vi "Example.vi"() -> ()   [LabVIEW 2016]
uses:
  Controls/Init_Parameters.ctl
  Controls/Error_Out.ctl
  Controls/ActorScalingDetailsLowT_Parameters.ctl
  Controls/ActorScalingDetailsRoomT_Parameters.ctl
  Controls/Frequency-Control_Parameters.ctl
  Controls/Actual-Value_Selection.ctl
  Controls/Invert-Polarity_Selection.ctl
  Controls/Amplitude-Control_Parameters.ctl
  Controls/Autoapproach_Parameters.ctl
  Controls/Stop-Condition-Autoapproach_Selection.ctl
  Controls/Autoapproach-Approach-Mode_Selection.ctl
  Controls/Autoapproach-Target-Mode_Selection.ctl
  Controls/Autoapproach-Details_Parameters.ctl
  Controls/Autoapproach-Axis_Selection.ctl
  Controls/Appraoch-Direction_Selection.ctl
  Controls/Autoapproach-Device_Selection.ctl
  Controls/Autoapproach-Trigger_Selection.ctl
  Controls/Ground-while-Appraoch_Selection.ctl
  Controls/DAC_Selection.ctl
  Controls/Generic-Feedback_Parameters.ctl
  Controls/Generic-Feedback-Number_Selection.ctl
  Controls/Generic-Feedback-Input-Channel_Selection.ctl
  Controls/Generic-Feedback-Output-Channel_Selection.ctl
  Controls/LF-Lockin_Parameters.ctl
  Controls/LF-Lockin-Output-Connector_Selection.ctl
  Controls/LF-Lockin-Input-Connector_Selection.ctl
  Controls/HF-Lockin_Parameters.ctl
  Controls/External-Transfer-Function_Parameters.ctl
  Controls/External-Transfer-Function_Selection.ctl
  Controls/External-Transfer-Function-Unit_Selection.ctl
  Controls/Dual-Pass_Parameters.ctl
  Controls/Dual-Pass-Alternative-Setpoint_Selection.ctl
  Controls/Dual-Pass-Alternative-DAC_Selection.ctl
  Controls/Dual-Pass-Alternative-Fexc_Selection.ctl
  Controls/Dual-Pass-Feedback-Mode_Selection.ctl
  Controls/Dual-Pass-State_Selection.ctl
  Controls/Scan_Parameters.ctl
  Controls/Spectroscopy_Parameters.ctl
  Controls/Spectroscopy-Mode_Selection.ctl
  Controls/Spec_DAC_Selection.ctl
  Controls/Channel_Parameters.ctl
  Controls/Channel_Selection.ctl
  Controls/Channel-Source_Selection.ctl
  Controls/Average_Selection.ctl
  Controls/Trigger_Selection.ctl
  Controls/Pathmode_Parameters.ctl
  Controls/Path-Mode-Edge_Selection.ctl
  Controls/Pathmode-Action_Selection.ctl
  Controls/Scanner_State_Machine.ctl
  Controls/DAC_Voltage.ctl
  Controls/DAC_Limits.ctl
  Controls/Z-Control_Parameters.ctl
  Controls/Coarse-Axis_Selection.ctl
  Controls/Grid_Parameters.ctl
  Controls/Output-Activation_Selection.ctl
panel:
  out "ScanUnits":string[](array[string])
  in  "Z Control Cluster":T1={"Input Signal"=0, "Min"=-inf, "Max"=-inf, "P"=-inf, "Setpoint a.u."=-inf, "Invert Polarity"=-2147483648, "I"=-inf} {"I" format="%#_g mHz"; "Invert Polarity" items=["[read only]"=-2147483648, "No"=0, "Yes"=1]; "Max" format="%#_g nm"; "Min" format="%#_g nm"; "Input Signal" items=["[read only]"=-2147483648, "ADC 1"=0, "ADC 2"=1, "ADC 3"=2, "ADC 4"=3, "ADC 5"=4, "ADC 6"=5, "HF 1 df"=8, "HF 1 Ampl"=13, "HF 1 Phase"=14, "LockIn Ampl"=16, "LockIn Phase"=17, "Counter"=23]}
  in  "Use sensor position":bool
  out "ErrCrt_Spec":bool
  out "ErrCrt_Line":bool
  out "storage paths":string[](array[string])
  in  "ScanStop":bool
  in  "Environment Temperature":sgl(slide)
  out "Enum":T4
  in  "Name of Profile":string="afm.ngp"
  in  "loop wait":u32=100 format="%.0f ms"
  out "unit_val 3":T5=-2147483648 items=["[read only]"=-2147483648, "Not Valid"=128, "m"=384, "mm"=383, "um"=382, "nm"=381, "pm"=380, "V"=640, "mV"=639, "uV"=638, "nV"=637, "MHz"=898, "kHz"=897, "Hz"=896, "mHz"=895, "Ks"=1153, "s"=1152, "ms"=1151, "us"=1150, "ns"=1149, "ps"=1148, "A"=1408, "mA"=1407, "uA"=1406, "nA"=1405, "W"=1664, "mW"=1663, "uW"=1662, "nW"=1661, "T"=1920, "mT"=1919, "uT"=1918, "nT"=1917, "K"=2176, "mK"=2175, "uK"=2174, "nK"=2173, "Deg"=2432, "mDeg"=2431, "uDeg"=2430, "nDeg"=2429, "[cos]"=2688, "[dB]"=2944, "LSB"=3200]
  out "unit_xy 3":T5=-2147483648 items=["[read only]"=-2147483648, "Not Valid"=128, "m"=384, "mm"=383, "um"=382, "nm"=381, "pm"=380, "V"=640, "mV"=639, "uV"=638, "nV"=637, "MHz"=898, "kHz"=897, "Hz"=896, "mHz"=895, "Ks"=1153, "s"=1152, "ms"=1151, "us"=1150, "ns"=1149, "ps"=1148, "A"=1408, "mA"=1407, "uA"=1406, "nA"=1405, "W"=1664, "mW"=1663, "uW"=1662, "nW"=1661, "T"=1920, "mT"=1919, "uT"=1918, "nT"=1917, "K"=2176, "mK"=2175, "uK"=2174, "nK"=2173, "Deg"=2432, "mDeg"=2431, "uDeg"=2430, "nDeg"=2429, "[cos]"=2688, "[dB]"=2944, "LSB"=3200]
  out "Intensity Graph":sgl[][](graph)
  out "ErrorStop":bool
  out "ErrCrt_Scan":bool
  out "unit_val":T5=-2147483648 items=["[read only]"=-2147483648, "Not Valid"=128, "m"=384, "mm"=383, "um"=382, "nm"=381, "pm"=380, "V"=640, "mV"=639, "uV"=638, "nV"=637, "MHz"=898, "kHz"=897, "Hz"=896, "mHz"=895, "Ks"=1153, "s"=1152, "ms"=1151, "us"=1150, "ns"=1149, "ps"=1148, "A"=1408, "mA"=1407, "uA"=1406, "nA"=1405, "W"=1664, "mW"=1663, "uW"=1662, "nW"=1661, "T"=1920, "mT"=1919, "uT"=1918, "nT"=1917, "K"=2176, "mK"=2175, "uK"=2174, "nK"=2173, "Deg"=2432, "mDeg"=2431, "uDeg"=2430, "nDeg"=2429, "[cos]"=2688, "[dB]"=2944, "LSB"=3200]
  out "unit_xy":T5=-2147483648 items=["[read only]"=-2147483648, "Not Valid"=128, "m"=384, "mm"=383, "um"=382, "nm"=381, "pm"=380, "V"=640, "mV"=639, "uV"=638, "nV"=637, "MHz"=898, "kHz"=897, "Hz"=896, "mHz"=895, "Ks"=1153, "s"=1152, "ms"=1151, "us"=1150, "ns"=1149, "ps"=1148, "A"=1408, "mA"=1407, "uA"=1406, "nA"=1405, "W"=1664, "mW"=1663, "uW"=1662, "nW"=1661, "T"=1920, "mT"=1919, "uT"=1918, "nT"=1917, "K"=2176, "mK"=2175, "uK"=2174, "nK"=2173, "Deg"=2432, "mDeg"=2431, "uDeg"=2430, "nDeg"=2429, "[cos]"=2688, "[dB]"=2944, "LSB"=3200]
  out "x != 0?":bool
  in  "Channel Cluster":T6={"Channel"=1, "Source"=-2147483648, "Average"=-2147483648, "SampleTime [us]"=-inf, "Trigger"=-2147483648} {"Trigger" items=["[read only]"=-2147483648, "Disabled"=0, "Scanner"=1, "Permanent"=2, "Spectroscopy 1"=3, "Spectroscopy 2"=4, "Spectroscopy 3"=5, "Calibration"=6, "Trigger"=7, "Every"=8, "Command"=9, "2nd Pass"=13, "Step Scan"=16]; "Average" items=["[read only]"=-2147483648, "no"=0, "yes"=1]; "Source" items=["[read only]"=-2147483648, "ADC 1"=0, "ADC 2"=1, "ADC 3"=2, "ADC 4"=3, "ADC 5"=4, "ADC 6"=5, "HF 1 Out"=7, "HF 1 df"=8, "z out"=9, "HF 1"=12, "HF 1 Ampl."=13, "HF 1 Phase"=14, "LF LockIn Ampl"=16, "LF LockIn Phase"=17, "z out inv"=18, "counter"=23, "Crosslink 1"=29, "Crosslink 2"=30, "Pos X"=31, "Pos Y"=32]; "Channel" items=["Channel 0", "Channel 1", "Channel 2", "Channel 3", "Channel 4", "Channel 5", "Channel 6", "Channel 7", "Channel 8", "Channel 9", "Channel 10", "Channel 11", "Channel 12", "Channel 13"]}
  in  "Corresponding channels":i32[](array[numeric])=[0, 1]
  in  "Output Status":bool
  out "Z out [nm]":sgl
  out "Z Pos Value":sgl(slide) min=0 max=40 scale=0.0..40.0
  in  "Start Feedback":bool
  in  "Retract":bool
  in  "Go to [nm]":sgl=-inf
  in  "Pause 2":bool caption="Pause"
  in  "SourceScan":u16(ring) items=["ADC 1", "ADC 2"]
  in  "Scan Parameters Cluster":T11={"Lines"=25, "Columns"=25, "X Range "=7503.493, "Y Range "=7503.493, "Pixel Size"=100.0, "Origin X"=3750.0, "Origin Y"=3750.0, "Rotation"=0.0, "Sample Time"=500.0} {"Sample Time" format="%#_g µs"; "Rotation" format="%#_g deg"; "Origin Y" format="%#_g nm"; "Origin X" format="%#_g nm"; "Pixel Size" format="%#_g nm"; "Y Range" format="%#_g nm"; "X Range" format="%#_g nm"; "Columns" max=250; "Lines" max=250}
  out "x-position":dbl format="%#_g µm"
  out "y-position":dbl format="%#_g µm"
  out "Scanner is":T12(ring)
  in  "Corresponding channels Scan":i32[](array[numeric])=[0, 1]
  in  "comment":string
  in  "binary":bool
  in  "Auto-save":bool
  out "Array":sgl[][][][](array[numeric])
  in  "fwd/bwd":bool=TRUE
  in  "Start Scan":bool
  in  "manual configuration":bool
  in  "Tab Control 2":enum32{"Line View", "Spectroscopy 1"}(tab)
  in  "Pause":bool
  out "Waveform Graph":sgl[](graph)
  in  "StopLine":bool
  in  "Displayed Data points":i32=5000 min=129
  in  "Source":T8 items=["[read only]"=-2147483648, "ADC 1"=0, "ADC 2"=1, "ADC 3"=2, "ADC 4"=3, "ADC 5"=4, "ADC 6"=5, "HF 1 Out"=7, "HF 1 df"=8, "z out"=9, "HF 1"=12, "HF 1 Ampl."=13, "HF 1 Phase"=14, "LF LockIn Ampl"=16, "LF LockIn Phase"=17, "z out inv"=18, "counter"=23, "Crosslink 1"=29, "Crosslink 2"=30, "Pos X"=31, "Pos Y"=32]
  in  "Save Button":bool
  out "XY Graph":cluster{sgl[], "specArrayY_bwd":sgl[]}[](graph)
  in  "SourceSpec":u16(ring)=3 items=["ADC 1"=3]
  in  "Spec Cluster":T13={"Mode"=0, "Start [a.u.]"=-inf, "End [a.u.]"=-inf, "Points"=-2147483648, "Repeat"=-2147483648, "Fwd/Bwd"=FALSE, "Delay"=-inf, "Preferences Button"=FALSE, "DAC"=0, "Avg Time"=-inf} {"Avg Time" format="%#_g µs"; "DAC" items=["DAC 1"=0, "DAC 2"=1, "DAC 3"=2, "DAC 4"=3, "Z"=26, "Low Frequency"=27]; "Delay" format="%#_g µs"; "Mode" items=["Spectroscopy 1", "Spectroscopy 2", "Spectroscopy 3", "Calibration"]}
  in  "Start Spectroscopy":bool
  out "error out":T16
  in  "Stop":bool
  in  "?":T17={"Path to server"="G:\\Development\\Share\\ELE\\_Projekte\\100xxx_ASC500_LabVIEW_Interface\\CurrentDaisySoftwareV27\\ASC500CL-18_10_11", "Server Host"=""}
  in  "Tab Control":T18(tab)
  in  "LT Input":T19={"x,y Max Voltage"=-inf, "x,y Max Range"=-inf, "z Max Voltage"=-inf, "z Max Range"=-inf} {"z Max Range" format="%#_g µm"; "z Max Voltage" format="%#_g V"; "x,y Max Range" format="%#_g µm"; "x,y Max Voltage" format="%#_g V"}
  in  "Set Details":bool
  in  "RT Input":T20={"xy Max Voltage"=-inf, "xy Max Range"=-inf, "z Max Voltage"=-inf, "z Max Range"=-inf} {"z Max Range" format="%#_g µm"; "z Max Voltage" format="%#_g V"; "xy Max Range" format="%#_g µm"; "xy Max Voltage" format="%#_g V"}
  in  "Frequency Control Cluster":T21={"Actual Value"=-2147483648, "Setpoint [a.u.]"=-inf, "Min"=-inf, "Invert Polarity"=-2147483648, "Max"=-inf, "df"=-inf, "P"=-inf, "f excite"=-inf, "I"=-inf, "state"=FALSE} {"I" format="%#_g mHz"; "f excite" format="%#_g kHz"; "df" format="%#_g kHz"; "Max" format="%#_g kHz"; "Invert Polarity" items=["[read only]"=-2147483648, "No"=0, "Yes"=1]; "Min" format="%#_g kHz"; "Actual Value" items=["[read only]"=-2147483648, "ADC 1"=0, "ADC 2"=1, "ADC 3"=2, "ADC 4"=3, "ADC 5"=4, "ADC 6"=5, "HF 1 df"=8, "HF 1 Ampl"=13, "HF 1 Phase"=14, "LockIn Ampl"=16, "LockIn Phase"=17, "Counter"=23]}
  in  "Amplitude Control":T22={"Amplitude"=-inf, "Min"=-inf, "Max"=-inf, "P"=-inf, "I"=-inf, "Setpoint"=-inf, "Invert Polarity"=-2147483648, "Loop"=FALSE} {"Invert Polarity" items=["[read only]"=-2147483648, "No"=0, "Yes"=1]; "Setpoint" format="%#_g V"; "I" format="%#_g Hz"; "Max" format="%#_g V"; "Min" format="%#_g V"; "Amplitude" format="%#_g V"}
  out "Actual df":sgl
  in  "autoapproach Cluster":T23={"Delay"=-inf, "Threshold [a.u.]"=-inf, "Stop Condition"=-2147483648, "Speed"=-inf, "Steps / Approach"=-2147483648, "Approach Mode"=-2147483648, "Target Mode"=-2147483648} {"Target Mode" items=["[read only]"=-2147483648, "Loop On"=0, "Retract"=1, "Loop Off"=2]; "Approach Mode" items=["[read only]"=-2147483648, "Ramp"=0, "Loop"=1]; "Speed" format="%#_g V/s"; "Stop Condition" items=["[read only]"=-2147483648, "> Threshold"=0, "< Threshold"=1]; "Delay" format="%#_g ms"}
  in  "Start AA":bool
  in  "Stop AA":bool
  in  "autoapproach details cluster":T27={"Axis"=-2147483648, "Direction"=-2147483648, "Device"=-2147483648, "Trigger Pol."=-2147483648, "Hold Time [us]"=-2147483648, "GND while Approach"=-2147483648} {"GND while Approach" items=["[read only]"=-2147483648, "No"=0, "Yes"=1]; "Trigger Pol." items=["[read only]"=-2147483648, "high active"=0, "low active"=1]; "Device" items=["[read only]"=-2147483648, "ANC300"=0, "TTL via DAC2"=1, "LVTTL via DAC2"=2, "ANC350 via NSL A"=3, "ANC350 via NSL B"=4, "attoSTM NSL A"=5, "attoSTM NSL B"=6]; "Direction" items=["[read only]"=-2147483648, "forward"=0, "backward"=1]; "Axis" items=["[read only]"=-2147483648, "Axis 1"=0, "Axis 2"=1, "Axis 3"=2]}
  out "Autoapproach Status":bool=TRUE
  out "HsReq":bool
  in  "Pathmode Cluster":T33={"Time [us]"=-inf, "Z Home [nm]"=-inf, "Edge"=-2147483648} {"Edge" items=["[read only]"=-2147483648, "Raising"=0, "Falling"=1]}
  in  "Define Grid":bool
  in  "Add To Path":bool
  in  "CoordX":sgl format="%#_g µm"
  in  "CoordY":sgl format="%#_g µm"
  in  "Stop Pathmode":bool
  in  "StartPathSinglePoints":bool
  in  "Add To Action List":bool
  in  "Action":T35 items=["Manual Handshake", "Z Spectroscopy", "DAC Spectroscopy", "Low Frequency Spectroscopy", "External Spectroscopy", "Move Z to Home", "Z Approach"]
  in  "Handshake":bool
  in  "Clear Path Mode Lists":bool
  in  "GridCluster":T36={"NumberOfPointsX"=2, "NumberOfPointsY"=3, "XCoordinates"=[0.0, 0.0, 0.0], "YCoordinates"=[0.0, 0.0, 0.0]} {"YCoordinates" format="%#_g µm"; "XCoordinates" format="%#_g µm"}
  in  "StartPathGrid":bool
  out "Actionlist":T35[](array[typedef]) items=["Manual Handshake", "Z Spectroscopy", "DAC Spectroscopy", "Low Frequency Spectroscopy", "External Spectroscopy", "Move Z to Home", "Z Approach"]
  out "PathPointList":string[][](table)
  in  "Make Steps":bool
  in  "Set Coarse":bool
  in  "Axis":T37 items=["Axis 1", "Axis 2", "Axis 3"]
  in  "NumberOfSteps\n(negativ for bwd)":i32=-2147483648
  in  "Coarse Input":T38 {"Amplitude" format="%.0f V"; "Frequency" format="%.0f Hz"}
  in  "Slewrate Value [V/s]":sgl=1.0
  in  "DAC":T39 items=["DAC 1", "DAC 2", "DAC 3", "DAC 4"]
  in  "Value [V]":T40=-inf format="%#_g V"
  in  "DAC-Limits":T41={"Current Limit"=-inf, "LT-Limit"=-inf, "RT-Limit"=-inf} {"RT-Limit" format="%#_g V"; "LT-Limit" format="%#_g V"; "Current Limit" format="%#_g V"}
  in  "Generic Tran Cluster":T42={"Number"=0, "P"=-inf, "Input Channel"=-2147483648, "I"=-2147483648, "Output Channel"=-2147483648, "Setpoint [a.u.]"=-inf, "Min"=-inf, "Invert Polarity"=-2147483648, "Max"=-inf, "Transfer function"=FALSE} {"Max" format="%#_g V"; "Invert Polarity" items=["[read only]"=-2147483648, "No"=0, "Yes"=1]; "Min" format="%#_g V"; "Output Channel" items=["[read only]"=-2147483648, "DAC 1"=0, "DAC 2"=1, "DAC 3"=2, "DAC 4"=3]; "I" format="%.0f mHz"; "Input Channel" items=["[read only]"=-2147483648, "ADC 1"=0, "ADC 2"=1, "ADC 3"=2, "ADC 4"=3, "ADC 5"=4, "ADC 6"=5, "HF 1 df "=8, "HF 1 Ampl"=13, "HF 1 Phase"=14, "LF LockIn Ampl"=16, "LF LockIn Phase"=17, "Counter"=23]; "Number" items=["1", "2"]}
  out "ActualGF":sgl
  in  "LF Lockin Cluster":T46={"Amplitude"=-inf, "Integration Time"=-inf, "Frequency"=-inf, "Output Connector"=-2147483648, "Sensitivity"=-inf, "Input Connector"=-2147483648, "Phase Shift"=-inf} {"Phase Shift" format="%#_g deg"; "Input Connector" items=["[read only]"=-2147483648, "ADC 1"=0, "ADC 2"=1, "ADC 3"=2, "ADC 4"=3, "ADC 5"=4, "ADC 6"=5, "SPM Z out"=9, "SPM Z out inv"=18, "AFM Signal"=12, "AFM df"=8, "AFM Aexc"=7, "AFM Aosc"=13, "AFM Phase"=14, "Lockin Ampl"=16, "Lockin Phase"=17]; "Sensitivity" format="%#_g V"; "Output Connector" items=["[read only]"=-2147483648, "Off"=0, "DAC 1"=1, "DAC 2"=2, "DAC 1 + DAC 2"=3]; "Frequency" format="%#_g kHz"; "Integration Time" format="%#_g µs"; "Amplitude" format="%#_g V"}
  in  "Feedback":sgl=-inf
  in  "Q Control":bool
  in  "HF Lockin Cluster":T49={"Amplitude"=-inf, "Phase Shift"=-inf, "Frequency"=-inf, "Integration Time"=-inf, "Sensitivity"=-inf} {"Sensitivity" format="%#_g V"; "Integration Time" format="%#_g µs"; "Frequency" format="%#_g kHz"; "Phase Shift" format="%#_g deg"; "Amplitude" format="%#_g V"}
  in  "Auto Phase":bool
  out "LF Amplitude":sgl format="%#_g V"
  out "LF Phase":sgl format="%#_g deg"
  out "HF Amplitude":sgl format="%#_g V"
  out "HF Phase":sgl format="%#_g deg"
  in  "Phase":sgl=-inf format="%#_g deg"
  in  "Exposure Time [us]":sgl=-inf
  in  "External Transfer Function Cluster":T50={"Number"=0, "Offset"=-inf, "Gain [Unit/V]"=-inf, "Unit"=-2147483648} {"Unit" items=["[read only]"=-2147483648, "Not Valid"=128, "m"=384, "mm"=383, "um"=382, "nm"=381, "pm"=380, "V"=640, "mV"=639, "uV"=638, "nV"=637, "MHz"=898, "kHz"=897, "Hz"=896, "mHz"=895, "Ks"=1153, "s"=1152, "ms"=1151, "us"=1150, "ns"=1149, "ps"=1148, "A"=1408, "mA"=1407, "uA"=1406, "nA"=1405, "W"=1664, "mW"=1663, "uW"=1662, "nW"=1661, "T"=1920, "mT"=1919, "uT"=1918, "nT"=1917, "K"=2176, "mK"=2175, "uK"=2174, "nK"=2173, "Deg"=2432, "mDeg"=2431, "uDeg"=2430, "nDeg"=2429, "[cos]"=2688, "[dB]"=2944, "LSB"=3200]; "Offset" format="%#_g mV"; "Number" items=["ADC 1", "ADC 2", "ADC 3", "ADC 4", "ADC 5", "ADC 6"]}
  in  "Dual Pass Cluster":T52={"Alternative Setpoint"=-2147483648, "Setpoint"=4.0, "Alternative DAC"=-2147483648, "Number of DAC"=1, "Value of DAC"=0, "Alternative Fexc"=-2147483648, "Value of Fexc"=10.0, "Lift Offset"=1000.0, "Wait Time"=5.0, "Lift Slewrate"=1.0} {"Lift Slewrate" format="%#_g V/s"; "Wait Time" format="%#_g ms"; "Lift Offset" format="%#_g nm"; "Value of Fexc" format="%#_g kHz"; "Alternative Fexc" items=["[read only]"=-2147483648, "No"=0, "Yes"=1]; "Value of DAC" format="%.0f V"; "Number of DAC" items=["DAC 1", "DAC 2", "DAC 3", "DAC 4"]; "Alternative DAC" items=["[read only]"=-2147483648, "No"=0, "Yes"=1]; "Alternative Setpoint" items=["[read only]"=-2147483648, "No"=0, "Yes"=1]}
  in  "Mode":T56=-2147483648 items=["[read only]"=-2147483648, "Feedback"=0, "First Line Profile"=1]
  in  "Enable dualpass":T57=-2147483648 items=["[read only]"=-2147483648, "No"=0, "Yes"=1]
  in  "gotoxy":bool
  in  "X":sgl format="%#_g µm"
  in  "Y":sgl format="%#_g µm"
  # "Z Control"
  # "Scan Parameters"
  # "Room Temp Input"
  # "Low Temp Input"
  # "Frequency Control"
  # "Amplitude Control"
  # "Autoapproach Parameters"
  # "Coarse"
  # "Generic Transfer Function"
  # "LF LockIn"
  # "HF LockIn"
  # "External Transfer Function"
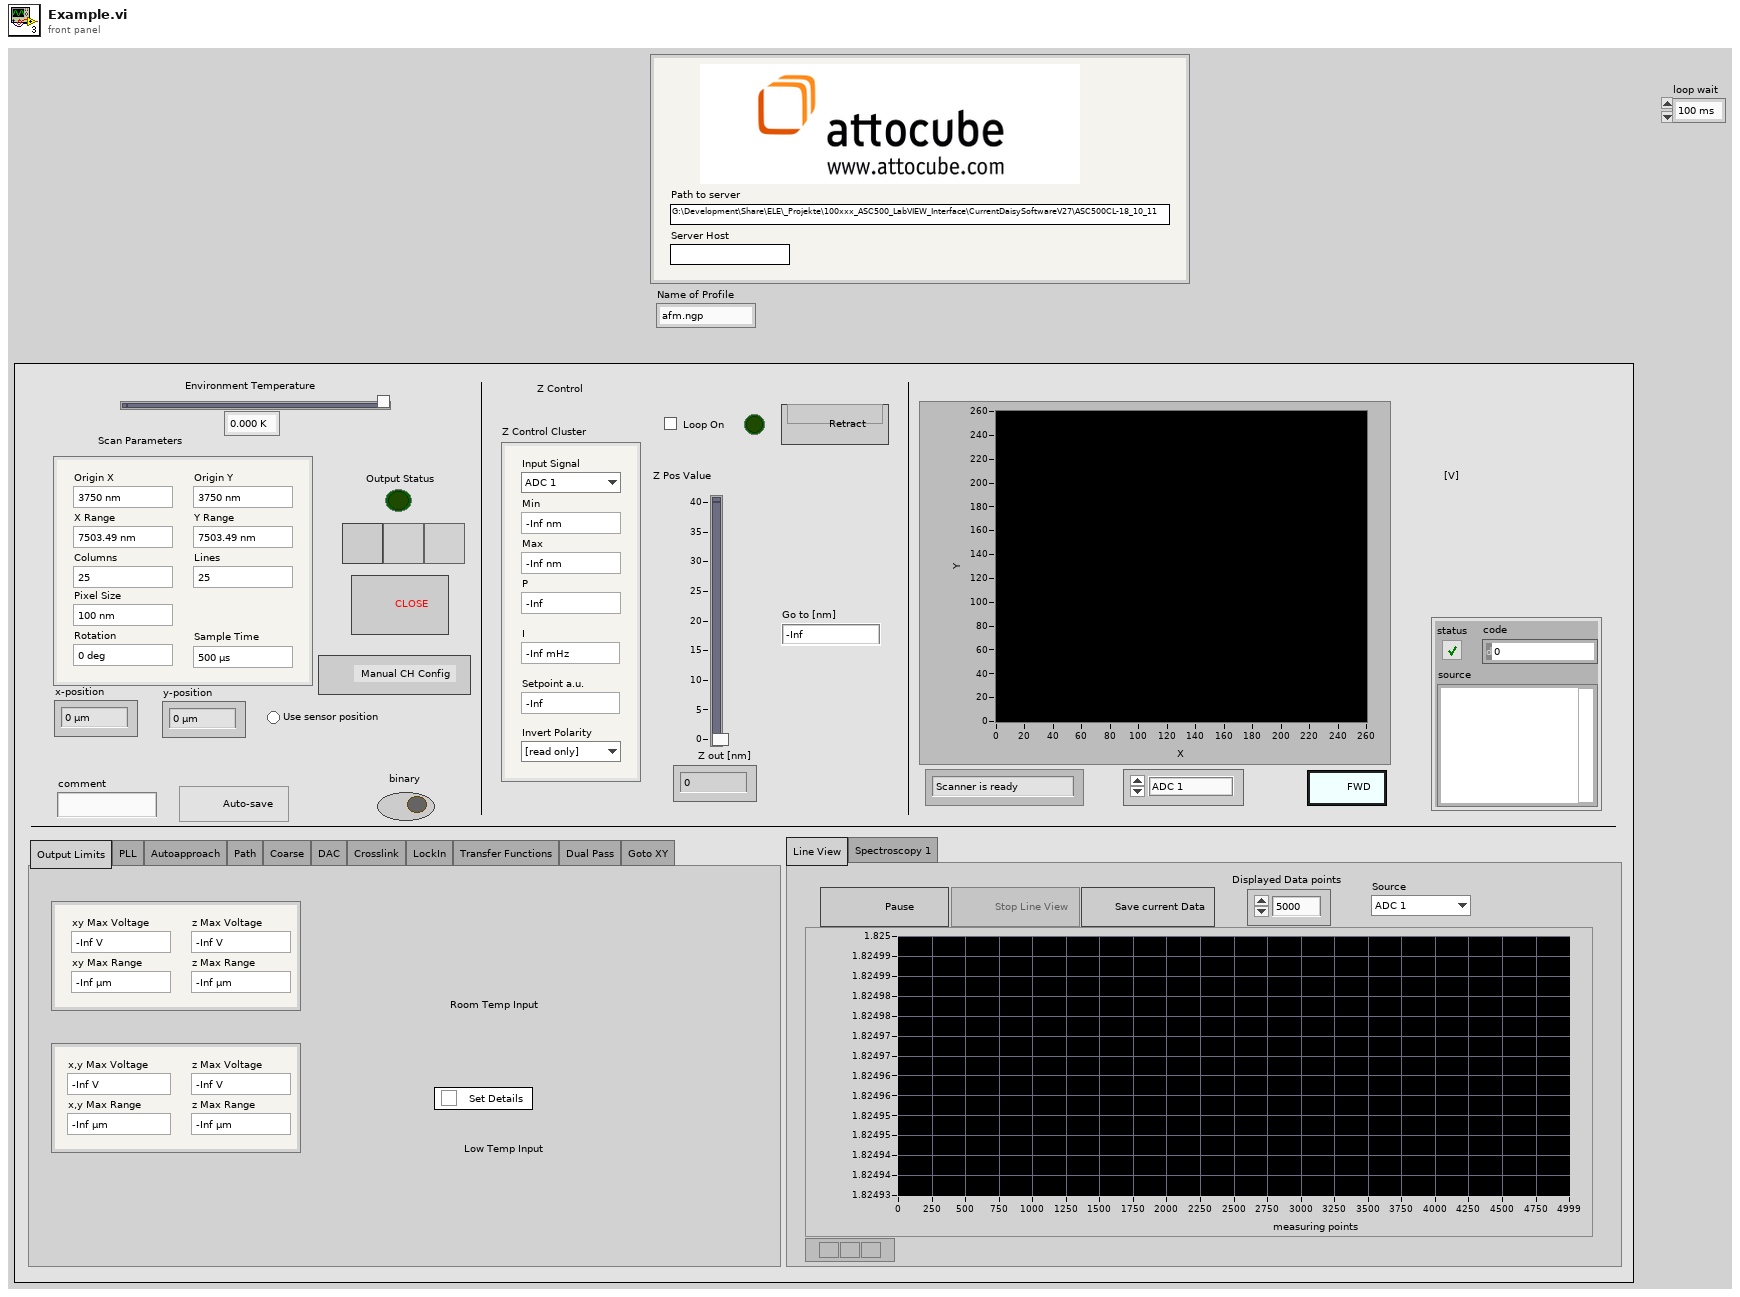
[diagram p1: front panel]
types:
  T1 = typedef "Z-Control_Parameters.ctl" = cluster{"Input Signal":T2, "Min":dbl, "Max":dbl, "P":dbl, "Setpoint a.u.":dbl, "Invert Polarity":T3, "I":dbl}
  T2 = typedef "Actual-Value_Selection.ctl" = i32
  T3 = typedef "Invert-Polarity_Selection.ctl" = i32
  T4 = typedef "Scanner_State_Machine.ctl" = enum16{"wait till start", "measure", "buffer data", "promt User", "save"}
  T5 = typedef "External-Transfer-Function-Unit_Selection.ctl" = i32
  T6 = typedef "Channel_Parameters.ctl" = cluster{"Channel":T7, "Source":T8, "Average":T9, "SampleTime [us]":sgl, "Trigger":T10}
  T7 = typedef "Channel_Selection.ctl" = i32
  T8 = typedef "Channel-Source_Selection.ctl" = i32
  T9 = typedef "Average_Selection.ctl" = i32
  T10 = typedef "Trigger_Selection.ctl" = i32
  T11 = typedef "Scan_Parameters.ctl" = cluster{"Lines":i32, "Columns":i32, "X Range ":sgl, "Y Range ":sgl, "Pixel Size":sgl, "Origin X":sgl, "Origin Y":sgl, "Rotation":sgl, "Sample Time":sgl}
  T12 = enum16{"Scanner is ready", "Scanner is running", "Scanner is paused", "Scanner is adjusting", "Scanner is returning to origin"}
  T13 = typedef "Spectroscopy_Parameters.ctl" = cluster{"Mode":T14, "Start [a.u.]":sgl, "End [a.u.]":sgl, "Points":i32, "Repeat":i32, "Fwd/Bwd":bool, "Delay":sgl, "Preferences Button":bool, "DAC":T15, "Avg Time":sgl}
  T14 = typedef "Spectroscopy-Mode_Selection.ctl" = u16
  T15 = typedef "Spec_DAC_Selection.ctl" = u16
  T16 = typedef "Error_Out.ctl" = errorcluster
  T17 = typedef "Init_Parameters.ctl" = cluster{"Path to server":string, "Server Host":string}
  T18 = enum32{"Output Limits", "PLL", "Autoapproach", "Path", "Coarse", "DAC", "Crosslink", "LockIn", "Transfer Functions", "Dual Pass", "Goto XY"}
  T19 = typedef "ActorScalingDetailsLowT_Parameters.ctl" = cluster{"x,y Max Voltage":dbl, "x,y Max Range":dbl, "z Max Voltage":dbl, "z Max Range":dbl}
  T20 = typedef "ActorScalingDetailsRoomT_Parameters.ctl" = cluster{"xy Max Voltage":dbl, "xy Max Range":dbl, "z Max Voltage":dbl, "z Max Range":dbl}
  T21 = typedef "Frequency-Control_Parameters.ctl" = cluster{"Actual Value":T2, "Setpoint [a.u.]":sgl, "Min":sgl, "Invert Polarity":T3, "Max":sgl, "df":sgl, "P":sgl, "f excite":sgl, "I":sgl, "state":bool}
  T22 = typedef "Amplitude-Control_Parameters.ctl" = cluster{"Amplitude":sgl, "Min":sgl, "Max":sgl, "P":sgl, "I":sgl, "Setpoint":sgl, "Invert Polarity":T3, "Loop":bool}
  T23 = typedef "Autoapproach_Parameters.ctl" = cluster{"Delay":sgl, "Threshold [a.u.]":sgl, "Stop Condition":T24, "Speed":sgl, "Steps / Approach":i32, "Approach Mode":T25, "Target Mode":T26}
  T24 = typedef "Stop-Condition-Autoapproach_Selection.ctl" = i32
  T25 = typedef "Autoapproach-Approach-Mode_Selection.ctl" = i32
  T26 = typedef "Autoapproach-Target-Mode_Selection.ctl" = i32
  T27 = typedef "Autoapproach-Details_Parameters.ctl" = cluster{"Axis":T28, "Direction":T29, "Device":T30, "Trigger Pol.":T31, "Hold Time [us]":i32, "GND while Approach":T32}
  T28 = typedef "Autoapproach-Axis_Selection.ctl" = i32
  T29 = typedef "Appraoch-Direction_Selection.ctl" = i32
  T30 = typedef "Autoapproach-Device_Selection.ctl" = i32
  T31 = typedef "Autoapproach-Trigger_Selection.ctl" = i32
  T32 = typedef "Ground-while-Appraoch_Selection.ctl" = i32
  T33 = typedef "Pathmode_Parameters.ctl" = cluster{"Time [us]":sgl, "Z Home [nm]":sgl, "Edge":T34}
  T34 = typedef "Path-Mode-Edge_Selection.ctl" = i32
  T35 = typedef "Pathmode-Action_Selection.ctl" = i32
  T36 = typedef "Grid_Parameters.ctl" = cluster{"NumberOfPointsX":i32, "NumberOfPointsY":i32, "XCoordinates":sgl[], "YCoordinates":sgl[]}
  T37 = typedef "Coarse-Axis_Selection.ctl" = u16
  T38 = cluster{"Axis":i32, "Frequency":i32, "Amplitude":i32}
  T39 = typedef "DAC_Selection.ctl" = u16
  T40 = typedef "DAC_Voltage.ctl" = sgl
  T41 = typedef "DAC_Limits.ctl" = cluster{"Current Limit":sgl, "LT-Limit":sgl, "RT-Limit":sgl}
  T42 = typedef "Generic-Feedback_Parameters.ctl" = cluster{"Number":T43, "P":sgl, "Input Channel":T44, "I":i32, "Output Channel":T45, "Setpoint [a.u.]":sgl, "Min":sgl, "Invert Polarity":T3, "Max":sgl, "Transfer function":bool}
  T43 = typedef "Generic-Feedback-Number_Selection.ctl" = i32
  T44 = typedef "Generic-Feedback-Input-Channel_Selection.ctl" = i32
  T45 = typedef "Generic-Feedback-Output-Channel_Selection.ctl" = i32
  T46 = typedef "LF-Lockin_Parameters.ctl" = cluster{"Amplitude":sgl, "Integration Time":sgl, "Frequency":sgl, "Output Connector":T47, "Sensitivity":sgl, "Input Connector":T48, "Phase Shift":sgl}
  T47 = typedef "LF-Lockin-Output-Connector_Selection.ctl" = i32
  T48 = typedef "LF-Lockin-Input-Connector_Selection.ctl" = i32
  T49 = typedef "HF-Lockin_Parameters.ctl" = cluster{"Amplitude":sgl, "Phase Shift":sgl, "Frequency":sgl, "Integration Time":sgl, "Sensitivity":sgl}
  T50 = typedef "External-Transfer-Function_Parameters.ctl" = cluster{"Number":T51, "Offset":sgl, "Gain [Unit/V]":dbl, "Unit":T5}
  T51 = typedef "External-Transfer-Function_Selection.ctl" = u16
  T52 = typedef "Dual-Pass_Parameters.ctl" = cluster{"Alternative Setpoint":T53, "Setpoint":sgl, "Alternative DAC":T54, "Number of DAC":T39, "Value of DAC":i32, "Alternative Fexc":T55, "Value of Fexc":sgl, "Lift Offset":sgl, "Wait Time":sgl, "Lift Slewrate":sgl}
  T53 = typedef "Dual-Pass-Alternative-Setpoint_Selection.ctl" = i32
  T54 = typedef "Dual-Pass-Alternative-DAC_Selection.ctl" = i32
  T55 = typedef "Dual-Pass-Alternative-Fexc_Selection.ctl" = i32
  T56 = typedef "Dual-Pass-Feedback-Mode_Selection.ctl" = i32
  T57 = typedef "Dual-Pass-State_Selection.ctl" = i32
  T58 = enum32{"Disabled", "Scan", "Line", "Spec 1", "Spec 2", "Spec 3", "Cal", "Trigger", "Every", "SoftSpec", "DualPass", "Step Scan"}
  T59 = typedef "Output-Activation_Selection.ctl" = i32
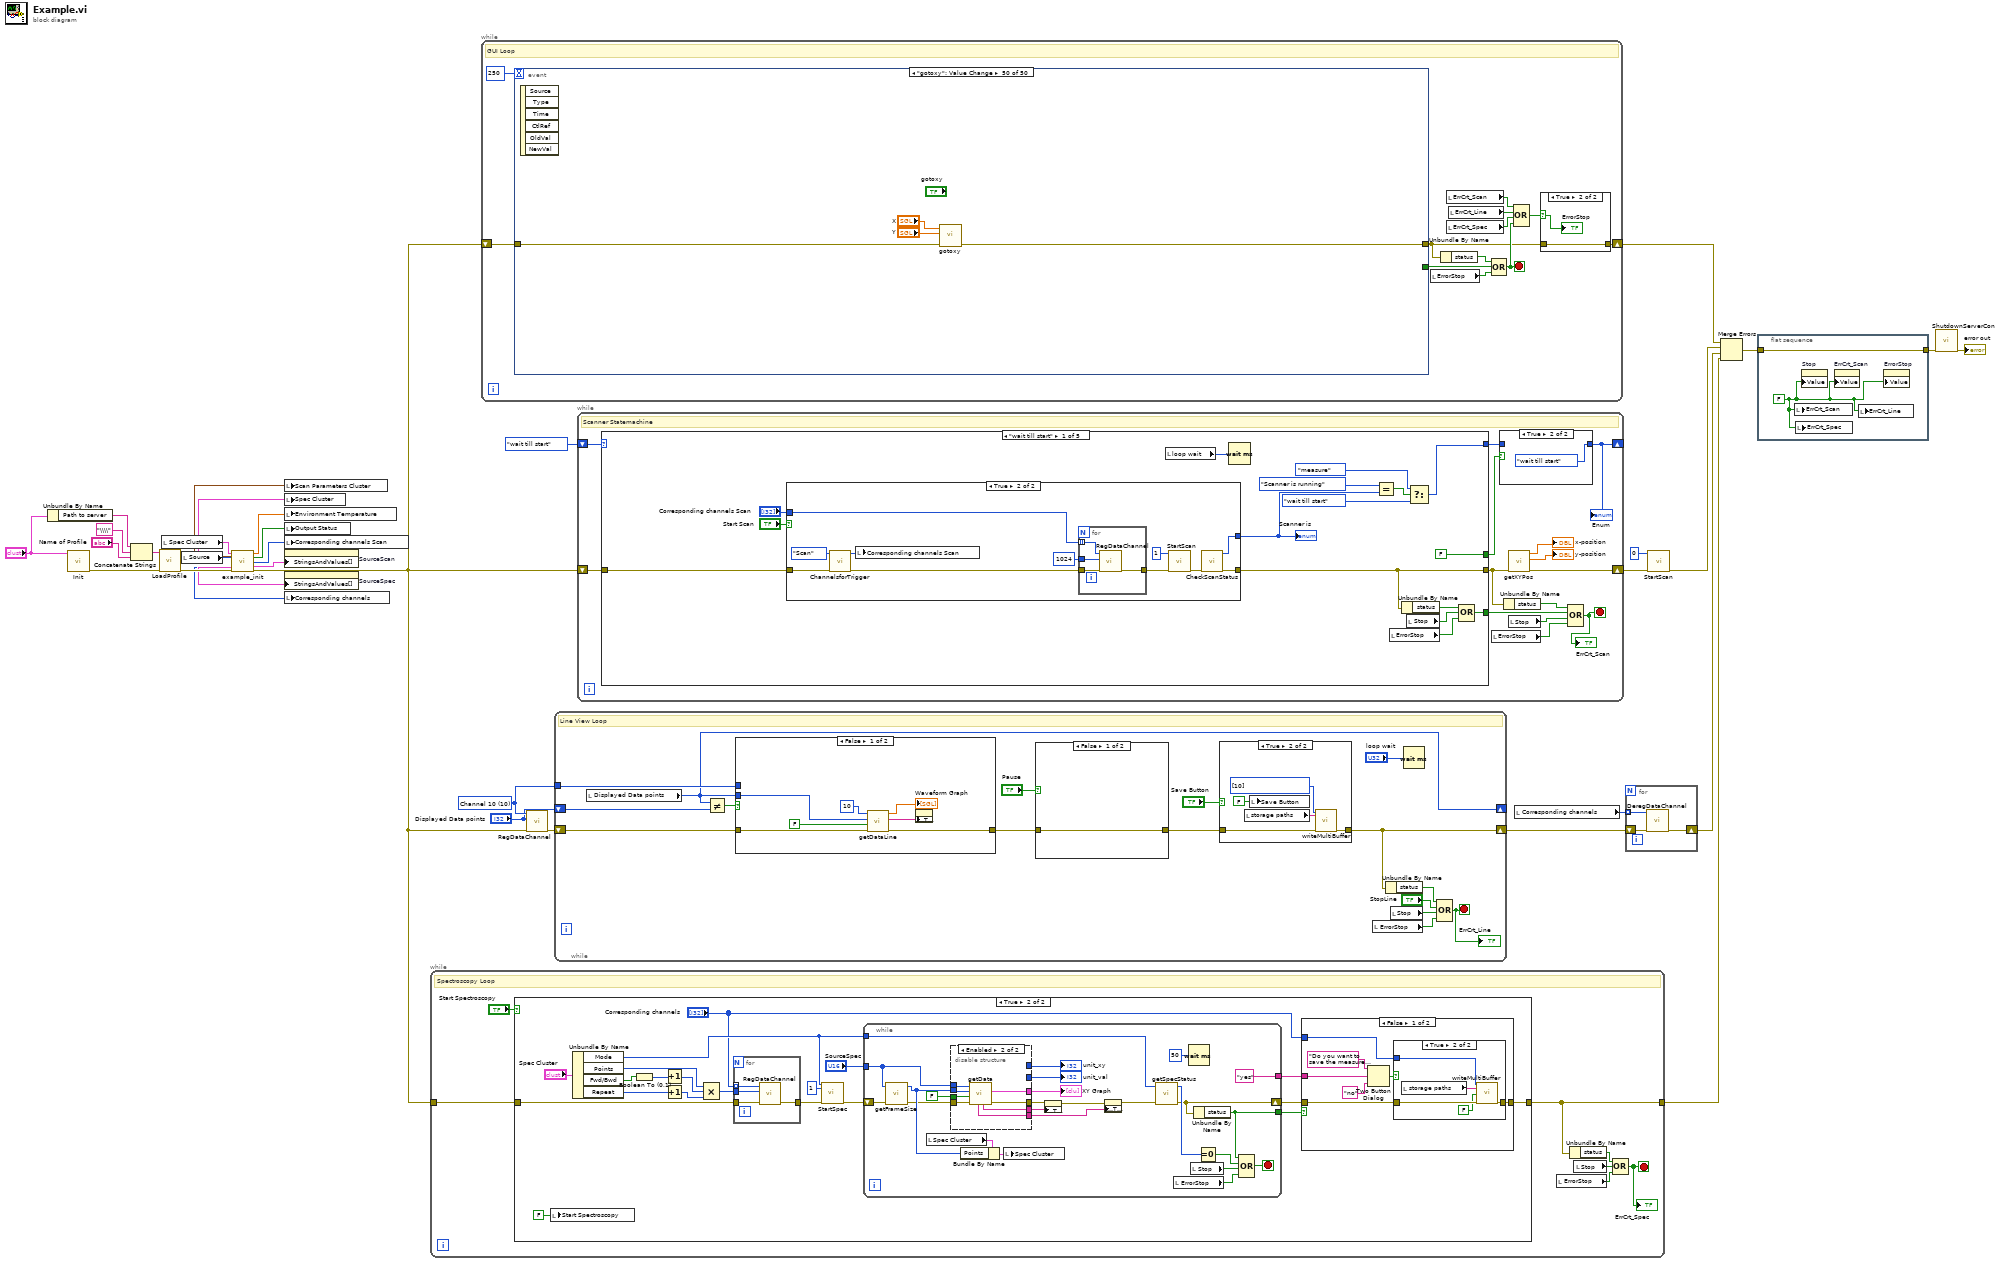
[diagram p0: block diagram]
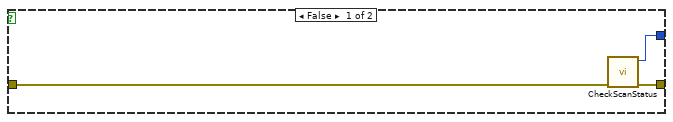
[diagram p3: hidden frame]
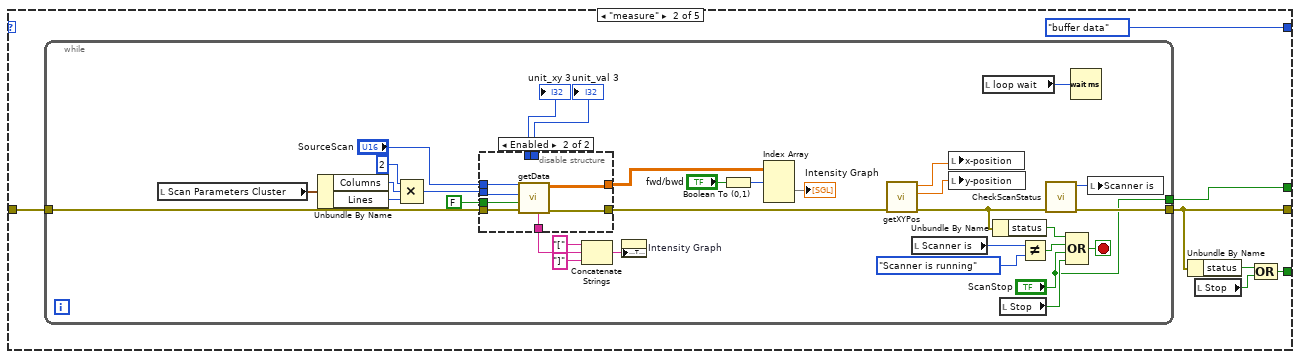
[diagram p4: hidden frame]
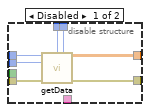
[diagram p5: hidden frame]
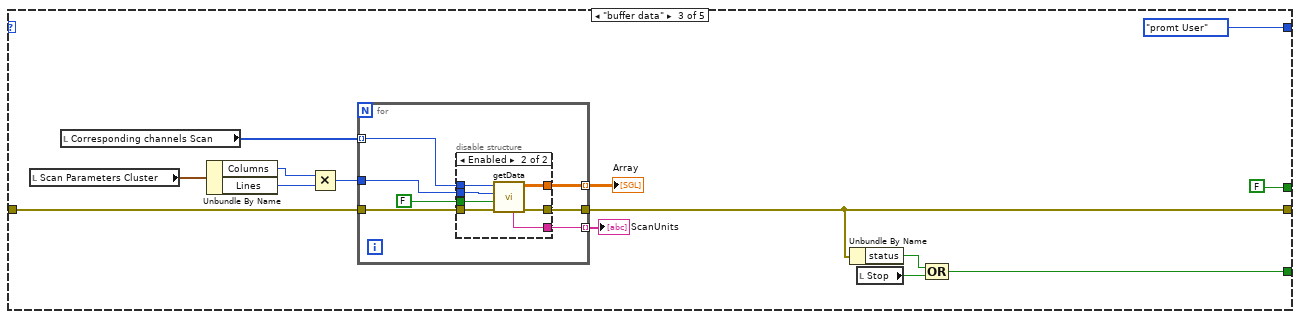
[diagram p6: hidden frame]
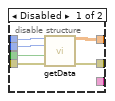
[diagram p7: hidden frame]
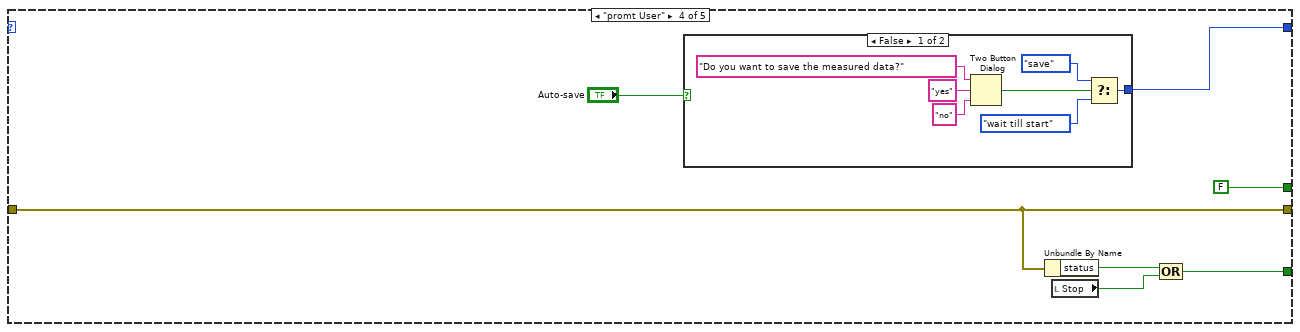
[diagram p8: hidden frame]
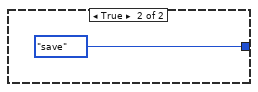
[diagram p9: hidden frame]
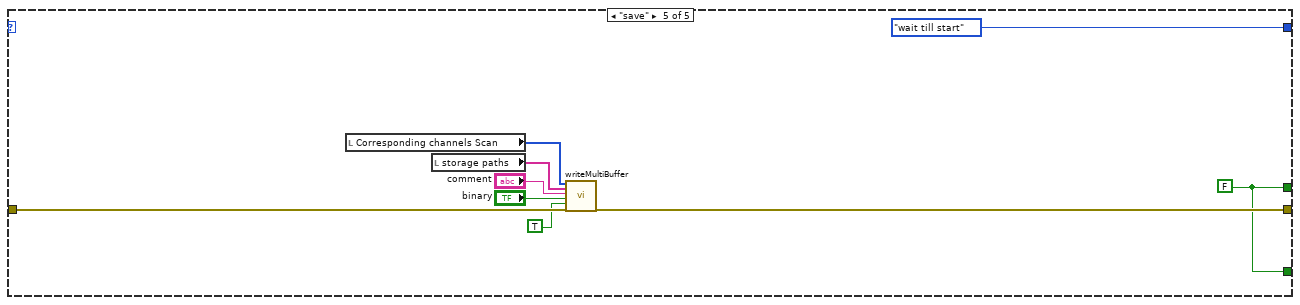
[diagram p10: hidden frame]
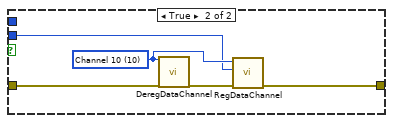
[diagram p12: hidden frame]
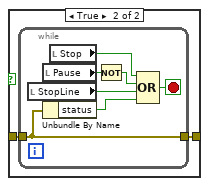
[diagram p13: hidden frame]
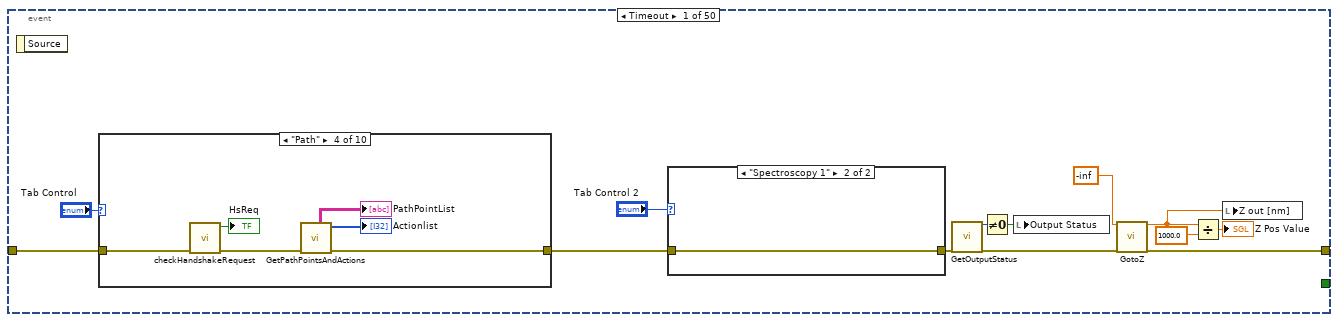
[diagram p15: hidden frame]
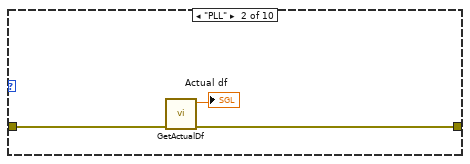
[diagram p18: hidden frame]
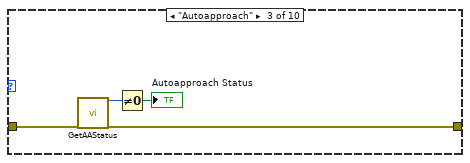
[diagram p19: hidden frame]
diagram:
  w10 = T7 10 items=["Channel 0", "Channel 1", "Channel 2", "Channel 3", "Channel 4", "Channel 5", "Channel 6", "Channel 7", "Channel 8", "Channel 9", "Channel 10", "Channel 11", "Channel 12", "Channel 13"] ("channel")
  n1 = Unbundle By Name("?") -> ("Path to server"=w27:string)
  n2 = call "Init.vi"("Init Cluster"="?") -> ("error out"=w15:T16)  [unwired: 10 in]
  n3 = Concatenate Strings(w27, "\\\\" ("path"), "Name of Profile") -> (w25:string)
  n4 = call "LoadProfile.vi"("path"=w25, "error in"=w15) -> ("error out"=w14:T16)  [unwired: 16 in, 1 out]
  n5 = local read "Spec Cluster"() -> (w23:T13)
  n6 = local read "Source"() -> (w21:T8)
  n7 = call "example_init.vi"("Spectroscopy Cluster"=w23, "Source for permanent"=w21, "error in"=w14) -> ("Scan Cluster"=w7:T11, "Spectroscopy Cluster"=w6:T13, "temperature"=w5:sgl, "Output Status"=w8:bool, "CorrespondingChScan"=w4:i32[], "SourceText_ChNumScan"=w22:cluster{"RingText.Text":string, i32}[], "CorrespondingChSpec"=w2:i32[], "SourceText_ChNumSpec"=w3:cluster{"RingText.Text":string, i32}[], "error out"=w1:T16)  [unwired: 4 in]
  n8 = local write "Scan Parameters Cluster"(w7) -> ()
  n9 = local write "Spec Cluster"(w6) -> ()
  n10 = local write "Environment Temperature"(w5) -> ()
  n11 = local write "Output Status"(w8) -> ()
  n12 = local write "Corresponding channels Scan"(w4) -> ()
  n13 = property on="SourceScan" class="Ring (strict)"("StringsAndValues[]"=w22) -> ()  [unwired: 2 in, 2 out]
  n14 = property on="SourceSpec" class="Ring (strict)"("StringsAndValues[]"=w3) -> ()  [unwired: 2 in, 2 out]
  n15 = local write "Corresponding channels"(w2) -> ()
  n16 = while {
    tunnel: [w36] -> w29
    tunnel: w1 -> [w37]
    stop <- w35 stop-if-true
    # "Spectroscopy Loop"
    n17 = case shown="True" "Start Spectroscopy" {
      tunnel: [w41 w51] -> w36
      tunnel: w37 -> [w41 w43]
      frame False {
        n18 = Wait (ms)(milliseconds to wait=u32 250) -> ()  [unwired: 1 out]
      }
      frame True {
        n19 = local write "Start Spectroscopy"(FALSE) -> ()
        n20 = Unbundle By Name("Spec Cluster") -> ("Mode"=w58:T14, "Points"=w57:i32, "Fwd/Bwd"=w55:bool, "Repeat"=w54:i32)
        n21 = Boolean To (0,1)(Boolean=w55) -> (0, 1=w56:i16)
        n22 = Increment(x=w56) -> (x+1=w44:i16)
        n23 = Increment(x=w54) -> (x+1=w53:i32)
        n24 = Compound Arithmetic op=MULTIPLY(w57, w44, w53) -> (w52:i32)
        n25 = for {
          tunnel: w43 -> [w118]
          tunnel: [w120] -> w61
          tunnel: "Corresponding channels" -> [w119] mode=indexing
          tunnel: w52 -> [w117]
          n26 = call "RegDataChannel.vi"("error in"=w118, "buffersize"=w117, "channel"=w119) -> ("error out"=w120:T16)  [unwired: 8 in]
        }
        n27 = call "StartSpec.vi"("Mode"=w58, "State"=1, "error in"=w61) -> ("error out"=w47:T16)  [unwired: 14 in, 2 out]
        n28 = while {
          tunnel: "SourceSpec" -> [w82]
          shift-right: [w87] -> w46
          shift-left: w47 -> [w94]
          tunnel: w58 -> [w99]
          tunnel: ["yes" ("T button name (\"OK\")")] -> w48
          tunnel: [w85] -> w45
          stop <- w101 stop-if-true
          n29 = call "getFrameSize.vi"("error in"=w94, "channel"=w82) -> ("error out"=w89:T16, "FrameSize"=w93:i32)  [unwired: 8 in]
          n30 = local read "Spec Cluster"() -> (w91:T13)
          n31 = disable-structure shown="Enabled" {
            disable-tunnel: [w108 _] -> w98
            disable-tunnel: [w107 _] -> w97
            disable-tunnel: [w106 w114] -> w96
            disable-tunnel: w82 -> [w105 w113]
            disable-tunnel: w93 -> [w104 w112]
            disable-tunnel: [w103 w115] -> w80
            disable-tunnel: w89 -> [w102 w116]
            disable-tunnel: FALSE ("fullOnly") -> [_ w111]
            disable-tunnel: [_ w110] -> w81
            disable-tunnel: [_ w109] -> w78
            frame Disabled {
              n32 = call "getData.vi"("Channel"=w105, "length"=w104, "error in"=w102) -> ("unit_xy"=w108:T5, "unit_val"=w107:T5, "Spec_Array"=w106:cluster{sgl[], "specArrayY_bwd":sgl[]}[], "error out"=w103:T16)  [unwired: 7 in, 2 out]
            }
            frame Enabled {
              n33 = call "getData.vi"("error in"=w116, "fullOnly"=w111, "length"=w112, "Channel"=w113) -> ("error out"=w115:T16, "Spec_Array"=w114:cluster{sgl[], "specArrayY_bwd":sgl[]}[], "unitStrVal"=w110:string, "unitStrXY"=w109:string)  [unwired: 3 in, 1 out]
            }
          }
          "XY Graph" <- w96
          "unit_xy" <- w98
          "unit_val" <- w97
          n34 = Bundle By Name(cluster=w91, "Points"=w93) -> (w92:T13)
          n35 = local write "Spec Cluster"(w92) -> ()
          n36 = property on="XY Graph" class="XYGraph (strict)"(error in=w80, "YScale.NameLbl.Text"=w81) -> (error out=w79:errorcluster)  [unwired: 1 in, 1 out]
          n37 = property on="XY Graph" class="XYGraph (strict)"(error in=w79, "XScale.NameLbl.Text"=w78) -> (error out=w77:errorcluster)  [unwired: 1 in, 1 out]
          n38 = call "getSpecStatus.vi"("error in"=w77, "index"=w99) -> ("error out"=w87:T16, "specstatus"=w95:i32)  [unwired: 8 in]
          n39 = local read "ErrorStop"() -> (w90:bool)
          n40 = Wait (ms)(milliseconds to wait=u32 50) -> ()  [unwired: 1 out]
          n41 = local read "Stop"() -> (w100:bool)
          n42 = Unbundle By Name(w87) -> ("status"=w85:bool)
          n43 = Equal To 0?(x=w95) -> (x = 0?=w86:bool)
          n44 = Compound Arithmetic op=OR(w85, w86, w100, w90) -> (w101:bool)
        }
        n45 = case shown="False" w45 {
          tunnel: [w69 w76] -> w51
          tunnel: "Corresponding channels" -> [w68 _]
          tunnel: w48 -> [w64 _]
          tunnel: w46 -> [w63 w76]
          frame False {
            n46 = Two Button Dialog(message="Do you want to save the measured data?", 1:"no" ("F button name (\"Cancel\")"), 2:w64) -> (T button?=w65:bool)
            n47 = case shown="True" w65 {
              tunnel: w63 -> [w70 w75]
              tunnel: [w70 w74] -> w69
              tunnel: w68 -> [_ w73]
              frame False {
              }
              frame True {
                n48 = local read "storage paths"() -> (w71:string[])
                n49 = call "writeMultiBuffer.vi"("Corresponding channels"=w73, "storage paths"=w71, "binary"=FALSE, "error in"=w75) -> ("error out"=w74:T16)  [unwired: 15 in]
              }
            }
          }
          frame True {
          }
        }
      }
    }
    n50 = local read "ErrorStop"() -> (w38:bool)
    n51 = Unbundle By Name(w36) -> ("status"=w39:bool)
    n52 = local read "Stop"() -> (w40:bool)
    n53 = Compound Arithmetic op=OR(w39, w40, w38) -> (w35:bool)
    "ErrCrt_Spec" <- w35
  }
  n54 = while {
    shift-right: [w121] -> w32
    shift-left: w1 -> [w132]
    stop <- w123 stop-if-true
    # "GUI Loop"
    n55 = event shown="[49] \"gotoxy\": Value Change" {
      selector: _ -> [_ _ _ _ _ _ _ _ _ _ _ _ _ _ _ _ _ _ _ _ _ _ _ _ _ _ _ _ _ _ _ _ _ _ _ _ _ _ _ _ _ _ _ _ _ _ _ _ _ _]
      dyn-events: _ -> [_ _ _ _ _ _ _ _ _ _ _ _ _ _ _ _ _ _ _ _ _ _ _ _ _ _ _ _ _ _ _ _ _ _ _ _ _ _ _ _ _ _ _ _ _ _ _ _ _ _]
      timeout: 250 -> [_ _ _ _ _ _ _ _ _ _ _ _ _ _ _ _ _ _ _ _ _ _ _ _ _ _ _ _ _ _ _ _ _ _ _ _ _ _ _ _ _ _ _ _ _ _ _ _ _ _]
      tunnel: [w147 w188 w192 w197 w210 w214 w216 w219 w222 w227 w231 w234 w241 w243 w248 w251 w257 w261 w265 w268 w271 w275 w278 w288 w301 w310 w315 w327 w345 w360 w377 w386 w389 w397 w399 w403 w409 w412 w416 w418 w422 w424 w427 w431 w434 w437 w442 w450 w456 w460] -> w122
      tunnel: w132 -> [w148 w188 w193 w202 w208 w212 w217 w220 w223 w228 w232 w235 w240 w244 w249 w252 w258 w262 w266 w269 w272 w276 w284 w289 w303 w311 w326 w331 w346 w361 w378 w388 w390 w398 w401 w404 w410 w413 w417 w419 w423 w425 w428 w432 w435 w438 w446 w451 w457 w461]
      tunnel: [_ TRUE _ _ _ _ _ _ _ _ _ _ _ _ _ _ _ _ _ _ _ _ _ _ _ _ _ _ _ _ _ _ _ _ _ _ _ _ _ _ _ _ _ _ _ _ _ _ _ _] -> w130
      event Timeout {
        n56 = event-data() -> ()  [unwired: 1 in, 1 out]
        n57 = case shown="\"Path\"" "Tab Control" {
          tunnel: w148 -> [w151 w153 w156 w164 w165 w171 w173 w185 w186 w187]
          tunnel: [w151 w152 w155 w162 w165 w169 w172 w181 w186 w187] -> w140
          frame "Output Limits", Default {
          }
          frame "PLL" {
            n58 = call "GetActualDf.vi"("error in"=w153) -> ("error out"=w152:T16, "Actual dF"=→"Actual df":sgl)  [unwired: 9 in]
          }
          frame "Autoapproach" {
            n59 = call "GetAAStatus.vi"("error in"=w156) -> ("State out"=w158:i32, "error out"=w155:T16)  [unwired: 17 in]
            n60 = Not Equal To 0?(x=w158) -> (x != 0?=→"Autoapproach Status":bool)
          }
          frame "Path" {
            n61 = call "checkHandshakeRequest.vi"("error in"=w164) -> ("error out"=w163:T16, "HsRequest"=→"HsReq":bool)  [unwired: 9 in]
            n62 = call "GetPathPointsAndActions.vi"("error in"=w163) -> ("error out"=w162:T16, "Actionlist"=→"Actionlist":T35[], "PathPoints"=→"PathPointList":string[][])  [unwired: 6 in, 2 out]
          }
          frame "Coarse" {
          }
          frame "DAC" {
            n63 = call "getDACLimits.vi"("error in"=w171, "DAC"="DAC") -> ("error out"=w170:T16, "DAC-Limits out"=w167:T41)  [unwired: 8 in]
            n64 = local write "DAC-Limits"(w167) -> ()
            n65 = call "GetDAC.vi"("Number of DAC"="DAC", "error in"=w170) -> ("DAC out"=w168:sgl, "error out"=w169:T16)  [unwired: 16 in]
            n66 = local write "Value [V]"(w168) -> ()
          }
          frame "Crosslink" {
            n67 = property on="Generic Tran Cluster" class="Clust (strict)"() -> ("Value"=w174:T42)  [unwired: 2 in, 2 out]
            n68 = Unbundle By Name(w174) -> ("Number"=w175:T43)
            n69 = call "GetActualGFOutput.vi"("Number"=w175, "error in"=w173) -> ("Value"=→"ActualGF":sgl, "error out"=w172:T16)  [unwired: 16 in]
          }
          frame "LockIn" {
            n70 = call "GetActLFLockInAmp.vi"("error in"=w185) -> ("Amplitude"=→"LF Amplitude":sgl, "error out"=w184:T16)  [unwired: 17 in]
            n71 = call "GetActLFLockInPhase.vi"("error in"=w184) -> ("Phase"=→"LF Phase":sgl, "error out"=w183:T16)  [unwired: 17 in]
            n72 = call "GetActHFLockInAmp.vi"("error in"=w183) -> ("Amplitude"=→"HF Amplitude":sgl, "error out"=w182:T16)  [unwired: 17 in]
            n73 = call "GetActHFLockInPhase.vi"("error in"=w182) -> ("Phase"=→"HF Phase":sgl, "error out"=w181:T16)  [unwired: 17 in]
          }
          frame "Transfer Functions" {
          }
          frame "Dual Pass" {
          }
        }
        n74 = case shown="\"Spectroscopy 1\"" "Tab Control 2" {
          tunnel: w140 -> [w149 w150]
          tunnel: [w149 w150] -> w139
          frame "Line View", Default {
          }
          frame "Spectroscopy 1" {
          }
        }
        n75 = call "GetOutputStatus.vi"("error in"=w139) -> ("Status out"=w144:i32, "error out"=w141:T16)  [unwired: 17 in]
        n76 = Not Equal To 0?(x=w144) -> (x != 0?=w142:bool)
        n77 = local write "Output Status"(w142) -> ()
        n78 = call "GotoZ.vi"("Z Target Pos"=sgl -inf ("Value [nm]"), "error in"=w141) -> ("Z Pos Out"=w145:sgl, "error out"=w147:T16)  [unwired: 16 in]
        n79 = Divide(x=w145, y=sgl 1000.0) -> (x/y=→"Z Pos Value":sgl)
        n80 = local write "Z out [nm]"(w145) -> ()
      }
      event "Stop": Value Change {
        n81 = event-data() -> ()  [unwired: 1 in, 1 out]
      }
      event "Environment Temperature": Value Change {
        n82 = event-data() -> ()  [unwired: 1 in, 6 out]
        n83 = call "SetActualTemperature.vi"("error in"=w193, "temperature in"="Environment Temperature") -> ("error out"=w192:T16, "temperature"=w190:sgl)  [unwired: 8 in]
        n84 = local write "Environment Temperature"(w190) -> ()
      }
      event "Set Details": Value Change {
        w199 = T59 1 items=["[read only]"=-2147483648, "off"=0, "on"=1] ("state")
        w203 = T59 0 items=["[read only]"=-2147483648, "off"=0, "on"=1] ("state")
        n85 = event-data() -> ()  [unwired: 1 in, 1 out]
        n86 = call "SetOutput.vi"("state"=w203, "error in"=w202) -> ("state out"=w200:T59, "error out"=w201:T16)  [unwired: 16 in]
        n87 = Not Equal To 0?(x=w200) -> (x != 0?=w194:bool)
        n88 = local write "Output Status"(w194) -> ()
        n89 = call "SetActorScalingDetailsLowT.vi"("error in"=w201, "Actor Scaling Details Low Temperature Input Cluster"="LT Input") -> ("error out"=w206:T16, "output cluster"=w195:T19)  [unwired: 8 in]
        n90 = local write "LT Input"(w195) -> ()
        n91 = call "SetActorScalingDetailsRoomT.vi"("error in"=w206, "Actor Scaling Details Room Temperature Input Cluster"="RT Input") -> ("error out"=w198:T16, "output cluster"=w196:T20)  [unwired: 8 in]
        n92 = local write "RT Input"(w196) -> ()
        n93 = call "SetOutput.vi"("state"=w199, "error in"=w198) -> ("error out"=w197:T16)  [unwired: 16 in, 1 out]
      }
      event Value Change {
        n94 = event-data() -> ()  [unwired: 1 in, 1 out]
        n95 = call "SetFrequencyControl.vi"("Frequency Control Cluster"="Frequency Control Cluster", "error in"=w208) -> ("Output Cluster"=w207:T21, "error out"=w210:T16)  [unwired: 16 in]
        n96 = local write "Frequency Control Cluster"(w207) -> ()
      }
      event Value Change {
        n97 = event-data() -> ()  [unwired: 1 in, 1 out]
        n98 = call "SetAmpControl.vi"("Amplitude Control Cluster"="Amplitude Control", "error in"=w212) -> ("Output Cluster"=w211:T22, "error out"=w214:T16)  [unwired: 16 in]
        n99 = local write "Amplitude Control"(w211) -> ()
      }
      event Value Change {
        n100 = event-data() -> ()  [unwired: 1 in, 1 out]
        n101 = call "SetAutoapproach.vi"("error in"=w217, "Autoapproach Cluster"="autoapproach Cluster") -> ("error out"=w216:T16, "Autoapproach Output"=w215:T23)  [unwired: 8 in]
        n102 = local write "autoapproach Cluster"(w215) -> ()
      }
      event "Start AA": Value Change {
        n103 = event-data() -> ()  [unwired: 1 in, 1 out]
        n104 = call "StartAA.vi"("State"=1, "error in"=w220) -> ("error out"=w219:T16)  [unwired: 16 in, 1 out]
      }
      event "Stop AA": Value Change {
        n105 = event-data() -> ()  [unwired: 1 in, 1 out]
        n106 = call "StartAA.vi"("State"=0, "error in"=w223) -> ("error out"=w222:T16)  [unwired: 16 in, 1 out]
      }
      event "Set Coarse": Value Change {
        n107 = event-data() -> ()  [unwired: 1 in, 1 out]
        n108 = call "SetCoarse.vi"("error in"=w228, "Coarse Input"="Coarse Input") -> ("error out"=w227:T16, "coarse output cluster"=w225:T38)  [unwired: 8 in]
        n109 = local write "Coarse Input"(w225) -> ()
      }
      event "Make Steps": Value Change {
        n110 = event-data() -> ()  [unwired: 1 in, 1 out]
        n111 = call "MakeSteps.vi"("Axis"="Axis", "Number"="NumberOfSteps\n(negativ for bwd)", "error in"=w232) -> ("error out"=w231:T16)  [unwired: 15 in, 1 out]
      }
      event Value Change {
        n112 = event-data() -> ()  [unwired: 1 in, 1 out]
        n113 = call "SetAutoapproachDetails.vi"("AA Details Cluster"="autoapproach details cluster", "error in"=w235) -> ("Output Cluster"=w233:T27, "error out"=w234:T16)  [unwired: 16 in]
        n114 = local write "autoapproach details cluster"(w233) -> ()
      }
      event Value Change {
        n115 = event-data() -> ()  [unwired: 1 in, 6 out]
        n116 = local read "DAC"() -> (w239:T39)
        n117 = call "SetDAC.vi"("error in"=w240, "Value [V]"="Value [V]", "Number"=w239) -> ("error out"=w241:T16, "Value"=w237:sgl)  [unwired: 6 in, 1 out]
        n118 = local write "Value [V]"(w237) -> ()
      }
      event "Slewrate Value [V/s]": Value Change {
        n119 = event-data() -> ()  [unwired: 1 in, 1 out]
        n120 = call "SetDACSlewrate.vi"("Value"="Slewrate Value [V/s]", "error in"=w244) -> ("Value out"=w242:sgl, "error out"=w243:T16)  [unwired: 16 in]
        n121 = local write "Slewrate Value [V/s]"(w242) -> ()
      }
      event Value Change {
        n122 = event-data() -> ()  [unwired: 1 in, 1 out]
        n123 = call "SetGenericFeedback.vi"("Generic Feedback Cluster"="Generic Tran Cluster", "error in"=w249) -> ("Output Cluster"=w246:T42, "error out"=w248:T16)  [unwired: 16 in]
        n124 = local write "Generic Tran Cluster"(w246) -> ()
      }
      event Value Change {
        n125 = event-data() -> ()  [unwired: 1 in, 1 out]
        n126 = call "SetLFLockIn.vi"("error in"=w252, "LF Lockin Cluster"="LF Lockin Cluster") -> ("error out"=w251:T16, "Output Cluster"=w250:T46)  [unwired: 8 in]
        n127 = local write "LF Lockin Cluster"(w250) -> ()
      }
      event "Feedback": Value Change {
        n128 = event-data() -> ()  [unwired: 1 in, 6 out]
        n129 = call "SetQControl.vi"("error in"=w258, "Feedback"="Feedback", "Phase"="Phase") -> ("error out"=w257:T16, "Feedback out"=w256:sgl, "Phase"=w254:sgl)  [unwired: 6 in]
        n130 = local write "Phase"(w254) -> ()
        n131 = local write "Feedback"(w256) -> ()
      }
      event "Q Control": Value Change {
        n132 = event-data() -> ()  [unwired: 1 in, 1 out]
        n133 = Boolean To (0,1)(Boolean="Q Control") -> (0, 1=w260:i16)
        n134 = call "StartQC.vi"("State"=w260, "error in"=w262) -> ("error out"=w261:T16)  [unwired: 16 in, 1 out]
      }
      event Value Change {
        n135 = event-data() -> ()  [unwired: 1 in, 1 out]
        n136 = call "SetHFLockIn.vi"("HF Lockin Cluster"="HF Lockin Cluster", "error in"=w266) -> ("Output Cluster"=w264:T49, "error out"=w265:T16)  [unwired: 16 in]
        n137 = local write "HF Lockin Cluster"(w264) -> ()
      }
      event "Auto Phase": Value Change {
        n138 = event-data() -> ()  [unwired: 1 in, 1 out]
        n139 = call "SetAutoPhase.vi"("error in"=w269) -> ("error out"=w268:T16)  [unwired: 18 in]
      }
      event "Exposure Time [us]": Value Change {
        n140 = event-data() -> ()  [unwired: 1 in, 1 out]
        n141 = call "SetExposureTime.vi"("Time"="Exposure Time [us]", "error in"=w272) -> ("Time out"=w270:sgl, "error out"=w271:T16)  [unwired: 16 in]
        n142 = local write "Exposure Time [us]"(w270) -> ()
      }
      event Value Change {
        n143 = event-data() -> ()  [unwired: 1 in, 1 out]
        n144 = call "SetExternalTransferFunction.vi"("Ext. Transfer Funct. Cluster"="External Transfer Function Cluster", "error in"=w276) -> ("Output Cluster"=w274:T50, "error out"=w275:T16)  [unwired: 16 in]
        n145 = local write "External Transfer Function Cluster"(w274) -> ()
      }
      event Value Change {
        n146 = event-data() -> ()  [unwired: 1 in, 6 out]
        n147 = call "SetZControl.vi"("Z Control Cluster"="Z Control Cluster", "error in"=w284) -> ("Z Control Output"=w279:T1, "error out"=w278:T16)  [unwired: 16 in]
        n148 = Unbundle By Name(w279) -> ("Max"=w282:dbl)
        n149 = local write "Z Control Cluster"(w279) -> ()
        n150 = Divide(x=w282, y=1000.0) -> (x/y=w281:dbl)
        n151 = property on="Z Pos Value" class="Slide (strict)"("Scale.Maximum"=w281) -> ()  [unwired: 2 in, 2 out]
      }
      event "Start Feedback": Value Change {
        n152 = event-data() -> ()  [unwired: 1 in, 1 out]
        n153 = case shown="False" "Start Feedback" {
          tunnel: w289 -> [w292 w296]
          tunnel: [w291 w295] -> w288
          tunnel: [w290 w294] -> w287
          frame False {
            n154 = call "StartFeedback.vi"("State"=0, "error in"=w292) -> ("State out"=w290:i32, "error out"=w291:T16)  [unwired: 16 in]
          }
          frame True {
            n155 = call "StartFeedback.vi"("State"=1, "error in"=w296) -> ("State out"=w294:i32, "error out"=w295:T16)  [unwired: 16 in]
          }
        }
        n156 = Not Equal To 0?(x=w287) -> (x != 0?=w285:bool)
        "x != 0?" <- w285
        n157 = local write "Start Feedback"(w285) -> ()
      }
      event "Retract": Value Change {
        n158 = event-data() -> ()  [unwired: 1 in, 6 out]
        n159 = disable-structure shown="Disabled" {
          disable-tunnel: w303 -> [w305 w306]
          disable-tunnel: [w304 w306] -> w302
          frame Disabled {
            n160 = call "Retract.vi"("error in"=w305) -> ("error out"=w304:T16)  [unwired: 18 in]
          }
          frame Enabled {
          }
        }
        n161 = call "StartFeedback.vi"("State"=0, "error in"=w302) -> ("State out"=w300:i32, "error out"=w301:T16)  [unwired: 16 in]
        n162 = Not Equal To 0?(x=w300) -> (x != 0?=w298:bool)
        n163 = local write "x != 0?"(w298) -> ()
        n164 = local write "Start Feedback"(w298) -> ()
      }
      event "Go to [nm]": Value Change {
        n165 = event-data() -> ()  [unwired: 1 in, 6 out]
        n166 = call "GotoZ.vi"("Z Target Pos"="Go to [nm]", "error in"=w311) -> ("Z Pos Out"=w308:sgl, "error out"=w310:T16)  [unwired: 16 in]
        "Z out [nm]" <- w308
        n167 = Divide(x=w308, y=sgl 1000.0) -> (x/y=w307:sgl)
        n168 = local write "Z Pos Value"(w307) -> ()
      }
      event "manual configuration": Value Change {
        n169 = event-data() -> ()  [unwired: 1 in, 1 out]
        n170 = call "manualChannelConfiguration.vi"("error in"=w326) -> ("error out"=w325:T16, "storage paths"=→"storage paths":string[])  [unwired: 9 in]
        n171 = call "getChannelConfig.vi"("error in"=w325, "Channel"=10) -> ("error out"=w317:T16, "source"=w324:i32)  [unwired: 5 in, 3 out]
        n172 = local write "Source"(w324) -> ()
        n173 = call "ChannelsforTrigger.vi"("Trigger"=T58."Scan", "error in"=w317) -> ("SourceText_ChNum"=w313:cluster{"RingText.Text":string, i32}[], "Corresponding channels"=w321:i32[], "error out"=w316:T16)  [unwired: 8 in, 3 out]
        n174 = property on="SourceScan" class="Ring (strict)"("StringsAndValues[]"=w313) -> ()  [unwired: 2 in, 2 out]
        n175 = local write "Corresponding channels Scan"(w321) -> ()
        n176 = call "ChannelsforTrigger.vi"("Trigger"=T58."Spec 1", "error in"=w316) -> ("SourceText_ChNum"=w318:cluster{"RingText.Text":string, i32}[], "Corresponding channels"=w319:i32[], "error out"=w315:T16)  [unwired: 8 in, 3 out]
        n177 = property on="SourceSpec" class="Ring (strict)"("StringsAndValues[]"=w318) -> ()  [unwired: 2 in, 2 out]
        n178 = local write "Corresponding channels"(w319) -> ()
      }
      event Value Change {
        n179 = event-data() -> ()  [unwired: 1 in, 1 out]
        n180 = call "CheckScanStatus.vi"("error in"=w331) -> ("error out"=w330:T16, "Scanner status"=w328:T12)  [unwired: 9 in]
        n181 = Equal To 0?(x=w328) -> (x = 0?=w329:bool)
        n182 = case shown="True" w329 {
          tunnel: w330 -> [w335 w340]
          tunnel: [w334 w339] -> w327
          frame False {
            n183 = call "setgetScanParameters.vi"("error in"=w335, "Set/Get"=FALSE) -> ("error out"=w334:T16, "Output Cluster"=w333:T11)  [unwired: 7 in, 1 out]
            n184 = local write "Scan Parameters Cluster"(w333) -> ()
            n185 = One Button Dialog(message="Scan parameters cannot be changed\nwhile scanner is running.", button name ("OK")="Ok") -> ()  [unwired: 1 out]
          }
          frame True {
            n186 = call "setgetScanParameters.vi"("error in"=w340, "Set/Get"=TRUE, "Scan Parameters Cluster"="Scan Parameters Cluster") -> ("error out"=w339:T16, "IN = OUT?"=w341:bool, "Output Cluster"=w342:T11)  [unwired: 6 in]
            n187 = case shown="False" w341 {
              tunnel: w342 -> [w344 _]
              frame False {
                n188 = local write "Scan Parameters Cluster"(w344) -> ()
              }
              frame True {
              }
            }
          }
        }
      }
      event "Start Scan": Value Change {
        n189 = event-data() -> ()  [unwired: 1 in, 1 out]
        n190 = while {
          shift-right: [w357] -> w345
          shift-left: w346 -> [w358]
          stop <- w350 stop-if-true
          n191 = call "CheckScanStatus.vi"("error in"=w358) -> ("error out"=w357:T16, "Scanner status"=w356:T12)  [unwired: 9 in]
          n192 = Equal?(x=w356, y=T12."Scanner is running" ("Scanner is 2")) -> (x = y?=w351:bool)
          n193 = local write "Scanner is"(w356) -> ()
          n194 = local read "ScanStop"() -> (w348:bool)
          n195 = local read "Stop"() -> (w349:bool)
          n196 = local read "Enum"() -> (w354:T4)
          n197 = Not Equal?(x=w354, y=Scanner_State_Machine."measure" ("Enum")) -> (x != y?=w352:bool)
          n198 = Wait (ms)(milliseconds to wait=u32 100) -> ()  [unwired: 1 out]
          n199 = Compound Arithmetic op=OR(w352, w351, w349, w348) -> (w350:bool)
        }
      }
      event "SourceScan", "fwd/bwd": Value Change {
        n200 = event-data() -> ()  [unwired: 1 in, 6 out]
        n201 = local read "Scanner is"() -> (w359:T12)
        n202 = Equal?(x=w359, y=T12."Scanner is ready" ("Scanner is 2")) -> (x = y?=w362:bool)
        n203 = case shown="True" w362 {
          tunnel: w361 -> [w364 w375]
          tunnel: [w364 w375] -> w360
          frame False {
          }
          frame True {
            n204 = local read "SourceScan"() -> (w369:u16)
            n205 = local read "fwd/bwd"() -> (w373:bool)
            n206 = local read "ScanUnits"() -> (w370:string[])
            n207 = local read "Array"() -> (w374:sgl[][][][])
            n208 = Not(x=w373) -> (.not. x?=w372:bool)
            n209 = Boolean To (0,1)(Boolean=w372) -> (0, 1=w376:i16)
            n210 = Index Array(array=w374, index (dim 0)=w369, index (dim 1)=w376) -> (element=w371:sgl[][])  [unwired: 2 in]
            n211 = Index Array(array=w370, index=w369) -> (element=w366:string)
            n212 = local write "Intensity Graph"(w371) -> ()
            n213 = Concatenate Strings("[", w366, "]") -> (w365:string)
            n214 = property on="Intensity Graph" class="IntGraph (strict)"("ZScale.NameLbl.Text"=w365) -> ()  [unwired: 2 in, 2 out]
          }
        }
      }
      event "Pause 2": Value Change {
        n215 = event-data() -> ()  [unwired: 1 in, 6 out]
        n216 = case shown="True" "Pause 2" {
          tunnel: w378 -> [w381 w385]
          tunnel: [w380 w384] -> w377
          frame False {
            n217 = call "StartScan.vi"("error in"=w381, "State"=1) -> ("error out"=w380:T16)  [unwired: 9 in]
          }
          frame True {
            n218 = call "StartScan.vi"("error in"=w385, "State"=2) -> ("error out"=w384:T16)  [unwired: 9 in]
          }
        }
      }
      event "ScanStop": Value Change {
        n219 = event-data() -> ()  [unwired: 1 in, 6 out]
        n220 = call "StartScan.vi"("error in"=w388, "State"=0) -> ("error out"=w386:T16)  [unwired: 9 in]
      }
      event Value Change {
        n221 = event-data() -> ()  [unwired: 1 in, 6 out]
        n222 = call "SetDualPass.vi"("Dual Pass Cluster"="Dual Pass Cluster", "error in"=w390) -> ("Output Cluster"=w394:T52, "error out"=w392:T16)  [unwired: 16 in]
        n223 = local write "Dual Pass Cluster"(w394) -> ()
        n224 = call "SetDualPassMode.vi"("Mode"="Mode", "error in"=w392) -> ("error out"=w389:T16)  [unwired: 16 in, 1 out]
      }
      event Value Change {
        n225 = event-data() -> ()  [unwired: 1 in, 6 out]
        n226 = call "EnableDualPass.vi"("error in"=w398, "Dual Pass State"="Enable dualpass") -> ("error out"=w397:T16, "Dual Pass State out"=w395:T57)  [unwired: 8 in]
        n227 = local write "Enable dualpass"(w395) -> ()
      }
      event Value Change {
        n228 = event-data() -> ()  [unwired: 1 in, 6 out]
        n229 = local read "Spec Cluster"() -> (w400:T13)
        n230 = call "SetSpecParameters.vi"("Spectroscopy Cluster"=w400, "error in"=w401) -> ("Output Cluster"=w402:T13, "error out"=w399:T16)  [unwired: 16 in]
        n231 = local write "Spec Cluster"(w402) -> ()
      }
      event Value Change {
        n232 = event-data() -> ()  [unwired: 1 in, 6 out]
        n233 = call "SetLimiterPopUp.vi"("error in"=w404) -> ("error out"=w403:T16)  [unwired: 10 in]
      }
      event Value Change {
        w405 = T7 10 items=["Channel 0", "Channel 1", "Channel 2", "Channel 3", "Channel 4", "Channel 5", "Channel 6", "Channel 7", "Channel 8", "Channel 9", "Channel 10", "Channel 11", "Channel 12", "Channel 13"] ("Channel")
        n234 = event-data() -> ()  [unwired: 1 in, 6 out]
        n235 = Bundle By Name(cluster="Channel Cluster", "Channel"=w405, "Source"="Source") -> (w407:T6)
        n236 = call "ConfigChannel.vi"("error in"=w410, "Channel Cluster"=w407) -> ("error out"=w409:T16)  [unwired: 8 in, 1 out]
      }
      event "Clear Path Mode Lists": Value Change {
        n237 = event-data() -> ()  [unwired: 1 in, 6 out]
        n238 = call "ClearPathModeLists.vi"("ClearActions"=1, "error in"=w413) -> ("error out"=w412:T16)  [unwired: 17 in]
      }
      event "Define Grid": Value Change {
        n239 = event-data() -> ()  [unwired: 1 in, 6 out]
        n240 = call "DefineGrid.vi"("error in"=w417, "Cluster"="GridCluster") -> ("error out"=w416:T16, "Output Cluster"=w414:T36)  [unwired: 8 in]
        n241 = local write "GridCluster"(w414) -> ()
      }
      event Value Change {
        n242 = event-data() -> ()  [unwired: 1 in, 6 out]
        n243 = call "SetPathmode.vi"("Pathmode Cluster"="Pathmode Cluster", "error in"=w419) -> ("Output Cluster"=w421:T33, "error out"=w418:T16)  [unwired: 16 in]
        n244 = local write "Pathmode Cluster"(w421) -> ()
      }
      event "Handshake": Value Change {
        n245 = event-data() -> ()  [unwired: 1 in, 6 out]
        n246 = call "Handshake.vi"("error in"=w423) -> ("error out"=w422:T16)  [unwired: 18 in]
      }
      event "Add To Action List": Value Change {
        n247 = event-data() -> ()  [unwired: 1 in, 6 out]
        n248 = call "AddToActionList.vi"("Action"="Action", "error in"=w425) -> ("error out"=w424:T16)  [unwired: 16 in, 1 out]
      }
      event "Add To Path": Value Change {
        n249 = event-data() -> ()  [unwired: 1 in, 6 out]
        n250 = call "AddPointToPath.vi"("error in"=w428, "CoordY"="CoordY", "CoordX"="CoordX") -> ("error out"=w427:T16)  [unwired: 7 in, 1 out]
      }
      event "StartPathSinglePoints": Value Change {
        n251 = event-data() -> ()  [unwired: 1 in, 6 out]
        n252 = call "StartPathMode.vi"("State"=1, "error in"=w432) -> ("error out"=w431:T16)  [unwired: 16 in, 1 out]
      }
      event "StartPathGrid": Value Change {
        n253 = event-data() -> ()  [unwired: 1 in, 6 out]
        n254 = call "StartPathMode.vi"("State"=2, "error in"=w435) -> ("error out"=w434:T16)  [unwired: 16 in, 1 out]
      }
      event "Stop Pathmode": Value Change {
        n255 = event-data() -> ()  [unwired: 1 in, 6 out]
        n256 = call "StartPathMode.vi"("State"=0, "error in"=w438) -> ("error out"=w437:T16)  [unwired: 16 in, 1 out]
      }
      event "Output Status": Value Change {
        n257 = event-data() -> ()  [unwired: 1 in, 6 out]
        n258 = Boolean To (0,1)(Boolean="Output Status") -> (0, 1=w444:i16)
        n259 = call "SetOutput.vi"("state"=w444, "error in"=w446) -> ("error out"=w443:T16)  [unwired: 16 in, 1 out]
        n260 = call "GetOutputStatus.vi"("error in"=w443) -> ("Status out"=w441:i32, "error out"=w442:T16)  [unwired: 17 in]
        n261 = Not Equal To 0?(x=w441) -> (x != 0?=w440:bool)
        n262 = local write "Output Status"(w440) -> ()
      }
      event Value Change {
        n263 = event-data() -> ()  [unwired: 1 in, 6 out]
        n264 = local read "DAC"() -> (w447:T39)
        n265 = call "setDACLimits.vi"("error in"=w451, "DAC"=w447, "DAC-Limits"="DAC-Limits") -> ("error out"=w450:T16, "DAC-Limits out"=w448:T41)  [unwired: 7 in]
        n266 = local write "DAC-Limits"(w448) -> ()
      }
      event "Use sensor position": Value Change {
        n267 = event-data() -> ()  [unwired: 1 in, 6 out]
        n268 = Boolean To (0,1)(Boolean="Use sensor position") -> (0, 1=w454:i16)
        n269 = call "setCLMode.vi"("error in"=w457, "CL-Mode"=w454) -> ("error out"=w456:T16, "CL-Mode out"=w452:i32)  [unwired: 8 in]
        n270 = Not Equal To 0?(x=w452) -> (x != 0?=w453:bool)
        n271 = local write "Use sensor position"(w453) -> ()
      }
      event "gotoxy": Value Change {
        n272 = event-data() -> ()  [unwired: 1 in, 6 out]
        n273 = call "gotoxy.vi"("error in"=w461, "yPos"="Y", "xPos"="X") -> ("error out"=w460:T16)  [unwired: 8 in]
      }
    }
    n274 = local read "ErrorStop"() -> (w128:bool)
    n275 = Unbundle By Name(w122) -> ("status"=w129:bool)
    n276 = local read "ErrCrt_Scan"() -> (w125:bool)
    n277 = local read "ErrCrt_Spec"() -> (w127:bool)
    n278 = local read "ErrCrt_Line"() -> (w126:bool)
    n279 = Compound Arithmetic op=OR(w129, w130, w128) -> (w123:bool)
    n280 = Compound Arithmetic op=OR(w125, w126, w127, w123) -> (w124:bool)
    n281 = case shown="True" w124 {
      selector: w124 -> [_ w135]
      tunnel: w122 -> [w133 w134]
      tunnel: [w133 w134] -> w121
      frame False {
      }
      frame True {
        "ErrorStop" <- w135
      }
    }
  }
  n282 = call "RegDataChannel.vi"("error in"=w1, "buffersize"="Displayed Data points", "channel"=w10) -> ("error out"=w11:T16)  [unwired: 8 in]
  n283 = while {
    shift-right: [w464] -> w13
    shift-left: w11 -> [w473]
    tunnel: w10 -> [w472]
    shift-right: [w467] -> _
    shift-left: "Displayed Data points" -> [w468]
    stop <- w462 stop-if-true
    # "Line View Loop"
    n284 = local read "Displayed Data points"() -> (w467:i32)
    n285 = Not Equal?(x=w467, y=w468) -> (x != y?=w469:bool)
    n286 = case shown="False" w469 {
      tunnel: w473 -> [w488 w494]
      tunnel: [w487 w492] -> w471
      tunnel: w467 -> [w489 w491]
      tunnel: w472 -> [_ _]
      frame False {
        n287 = call "getDataLine.vi"("error in"=w488, "FullOnly"=FALSE, "length"=w489, "channel"=10) -> ("error out"=w487:T16, "Unit value"=w484:string, "linearray"=→"Waveform Graph":sgl[])  [unwired: 5 in]
        n288 = property on="Waveform Graph" class="WFGraph (strict)"("YScale.NameLbl.Text"=w484) -> ()  [unwired: 2 in, 2 out]
      }
      frame True {
        w495 = T7 10 items=["Channel 0", "Channel 1", "Channel 2", "Channel 3", "Channel 4", "Channel 5", "Channel 6", "Channel 7", "Channel 8", "Channel 9", "Channel 10", "Channel 11", "Channel 12", "Channel 13"] ("channel")
        n289 = call "DeregDataChannel.vi"("channel"=w495, "error in"=w494) -> ("error out"=w493:T16)  [unwired: 17 in]
        n290 = call "RegDataChannel.vi"("error in"=w493, "buffersize"=w491, "channel"=w495) -> ("error out"=w492:T16)  [unwired: 8 in]
      }
    }
    n291 = case shown="False" "Pause" {
      tunnel: w471 -> [w496 w498]
      tunnel: [w496 w497] -> w465
      frame False {
      }
      frame True {
        n292 = while {
          tunnel: w498 -> [w505]
          tunnel: [w505] -> w497
          stop <- w503 stop-if-true
          n293 = local read "StopLine"() -> (w500:bool)
          n294 = local read "Pause"() -> (w501:bool)
          n295 = Unbundle By Name(w505) -> ("status"=w504:bool)
          n296 = local read "Stop"() -> (w499:bool)
          n297 = Not(x=w501) -> (.not. x?=w502:bool)
          n298 = Compound Arithmetic op=OR(w499, w502, w500, w504) -> (w503:bool)
        }
      }
    }
    n299 = case shown="True" "Save Button" {
      tunnel: [w478 w482] -> w464
      tunnel: w465 -> [w478 w483]
      frame False {
      }
      frame True {
        w481 = T7[] [10] items=["Channel 0", "Channel 1", "Channel 2", "Channel 3", "Channel 4", "Channel 5", "Channel 6", "Channel 7", "Channel 8", "Channel 9", "Channel 10", "Channel 11", "Channel 12", "Channel 13"]
        n300 = local read "storage paths"() -> (w479:string[])
        n301 = local write "Save Button"(FALSE ("Save Button")) -> ()
        n302 = call "writeMultiBuffer.vi"("Corresponding channels"=w481, "storage paths"=w479, "error in"=w483) -> ("error out"=w482:T16)  [unwired: 16 in]
      }
    }
    n303 = local read "ErrorStop"() -> (w466:bool)
    n304 = Unbundle By Name(w464) -> ("status"=w477:bool)
    n305 = local read "Stop"() -> (w474:bool)
    n306 = Wait (ms)(milliseconds to wait="loop wait") -> ()  [unwired: 1 out]
    n307 = Compound Arithmetic op=OR(w477, "StopLine", w474, w466) -> (w462:bool)
    "ErrCrt_Line" <- w462
  }
  n308 = while {
    shift-right: [w515] -> _
    shift-left: Scanner_State_Machine."wait till start" ("Enum") -> [w518]
    shift-right: [w506] -> w19
    shift-left: w1 -> [w519]
    stop <- w509 stop-if-true
    # "Scanner Statemachine"
    n309 = case shown="\"wait till start\"" w518 {
      tunnel: [w530 Scanner_State_Machine."buffer data" ("Enum") Scanner_State_Machine."promt User" ("Enum 2") w649 Scanner_State_Machine."wait till start" ("Enum 2")] -> w516
      tunnel: w519 -> [w527 w560 w622 w643 w665]
      tunnel: [w526 w562 w621 w643 w664] -> w512
      tunnel: [FALSE ("Stop 2") w559 FALSE FALSE ("Stop 2") w661] -> w514
      tunnel: [w529 w556 w611 w644 w661] -> w513
      frame "wait till start" {
        n310 = case shown="True" "Start Scan" {
          tunnel: [w540 w543] -> w528
          tunnel: w527 -> [w539 w545]
          tunnel: [w538 w544] -> w526
          tunnel: "Corresponding channels Scan" -> [_ w542]
          frame False {
            n311 = call "CheckScanStatus.vi"("error in"=w539) -> ("error out"=w538:T16, "Scanner status"=w540:T12)  [unwired: 9 in]
          }
          frame True {
            n312 = call "ChannelsforTrigger.vi"("Trigger"=T58."Scan", "error in"=w545) -> ("Corresponding channels"=w546:i32[], "error out"=w550:T16)  [unwired: 8 in, 4 out]
            n313 = local write "Corresponding channels Scan"(w546) -> ()
            n314 = for {
              tunnel: [w555] -> w551
              tunnel: 1024 ("value") -> [w554]
              tunnel: w550 -> [w553]
              tunnel: w542 -> [w552] mode=indexing
              n315 = call "RegDataChannel.vi"("error in"=w553, "buffersize"=w554, "channel"=w552) -> ("error out"=w555:T16)  [unwired: 8 in]
            }
            n316 = call "StartScan.vi"("error in"=w551, "State"=1) -> ("error out"=w549:T16)  [unwired: 9 in]
            n317 = call "CheckScanStatus.vi"("error in"=w549) -> ("error out"=w544:T16, "Scanner status"=w543:T12)  [unwired: 9 in]
          }
        }
        "Scanner is" <- w528
        n318 = local read "loop wait"() -> (w522:u32)
        n319 = Wait (ms)(milliseconds to wait=w522) -> ()  [unwired: 1 out]
        n320 = Equal?(x=T12."Scanner is running" ("Scanner is"), y=w528) -> (x = y?=w531:bool)
        n321 = local read "ErrorStop"() -> (w523:bool)
        n322 = Unbundle By Name(w526) -> ("status"=w537:bool)
        n323 = local read "Stop"() -> (w536:bool)
        n324 = Select(t=Scanner_State_Machine."measure" ("Enum"), s=w531, f=Scanner_State_Machine."wait till start" ("Enum")) -> (s? t:f=w530:T4)
        n325 = Compound Arithmetic op=OR(w537, w536, w523) -> (w529:bool)
      }
      frame "measure" {
        n326 = while {
          tunnel: w560 -> [w576]
          tunnel: [w587] -> w562
          tunnel: ["ScanStop"] -> w559
          stop <- w591 stop-if-true
          n327 = local read "Scan Parameters Cluster"() -> (w585:T11)
          n328 = Unbundle By Name(w585) -> ("Columns"=w571:i32, "Lines"=w583:i32)
          n329 = Compound Arithmetic op=MULTIPLY(2 ("value"), w571, w583) -> (w580:i32)
          n330 = disable-structure shown="Enabled" {
            disable-tunnel: [w601 w607] -> w589
            disable-tunnel: [w600 _] -> w582
            disable-tunnel: [w599 _] -> w581
            disable-tunnel: w580 -> [w598 w606]
            disable-tunnel: w576 -> [w597 w608]
            disable-tunnel: "SourceScan" -> [w596 w605]
            disable-tunnel: [w595 w604] -> w573
            disable-tunnel: FALSE ("fullOnly") -> [_ w603]
            disable-tunnel: [_ w602] -> w566
            frame Disabled {
              n331 = call "getData.vi"("Channel"=w596, "length"=w598, "error in"=w597) -> ("unit_xy"=w600:T5, "unit_val"=w599:T5, "scanData"=w595:sgl[][][], "error out"=w601:T16)  [unwired: 7 in, 2 out]
            }
            frame Enabled {
              n332 = call "getData.vi"("error in"=w608, "fullOnly"=w603, "length"=w606, "Channel"=w605) -> ("error out"=w607:T16, "scanData"=w604:sgl[][][], "unitStrVal"=w602:string)  [unwired: 3 in, 2 out]
            }
          }
          "unit_xy 3" <- w582
          "unit_val 3" <- w581
          n333 = Concatenate Strings("[", w566, "]") -> (w563:string)
          n334 = property on="Intensity Graph" class="IntGraph (strict)"("ZScale.NameLbl.Text"=w563) -> ()  [unwired: 2 in, 2 out]
          n335 = Boolean To (0,1)(Boolean="fwd/bwd") -> (0, 1=w578:i16)
          n336 = Index Array(array=w573, index (dim 0)=w578) -> (element=→"Intensity Graph":sgl[][])  [unwired: 2 in]
          n337 = call "getXYPos.vi"("error in"=w589) -> ("error out"=w588:T16, "y"=w568:dbl, "x"=w569:dbl)  [unwired: 8 in]
          n338 = local read "Scanner is"() -> (w594:T12)
          n339 = local write "x-position"(w569) -> ()
          n340 = local write "y-position"(w568) -> ()
          n341 = local read "loop wait"() -> (w572:u32)
          n342 = Unbundle By Name(w588) -> ("status"=w593:bool)
          n343 = local read "Stop"() -> (w584:bool)
          n344 = Not Equal?(x=w594, y=T12."Scanner is running" ("Scanner is 2")) -> (x != y?=w592:bool)
          n345 = call "CheckScanStatus.vi"("error in"=w588) -> ("error out"=w587:T16, "Scanner status"=w586:T12)  [unwired: 9 in]
          n346 = Compound Arithmetic op=OR(w593, w592, "ScanStop", w584) -> (w591:bool)
          n347 = Wait (ms)(milliseconds to wait=w572) -> ()  [unwired: 1 out]
          n348 = local write "Scanner is"(w586) -> ()
        }
        n349 = Unbundle By Name(w562) -> ("status"=w558:bool)
        n350 = local read "Stop"() -> (w557:bool)
        n351 = Compound Arithmetic op=OR(w558, w557) -> (w556:bool)
      }
      frame "buffer data" {
        n352 = local read "Scan Parameters Cluster"() -> (w619:T11)
        n353 = local read "Corresponding channels Scan"() -> (w610:i32[])
        n354 = Unbundle By Name(w619) -> ("Columns"=w618:i32, "Lines"=w617:i32)
        n355 = Multiply(x=w618, y=w617) -> (x*y=w616:i32)
        n356 = for {
          tunnel: w622 -> [w629]
          tunnel: [w628] -> w621
          tunnel: w610 -> [w627] mode=indexing
          tunnel: [w624] -> w612 mode=indexing
          tunnel: w616 -> [w625]
          tunnel: [w623] -> w609 mode=indexing
          n357 = disable-structure shown="Enabled" {
            disable-tunnel: w629 -> [w635 w640]
            disable-tunnel: [w634 w639] -> w628
            disable-tunnel: w627 -> [w633 w642]
            disable-tunnel: FALSE -> [w632 w637]
            disable-tunnel: w625 -> [w631 w641]
            disable-tunnel: [w630 w638] -> w624
            disable-tunnel: [_ w636] -> w623
            frame Disabled {
              n358 = call "getData.vi"("Channel"=w633, "length"=w631, "error in"=w635, "fullOnly"=w632) -> ("scanData"=w630:sgl[][][], "error out"=w634:T16)  [unwired: 6 in, 4 out]
            }
            frame Enabled {
              n359 = call "getData.vi"("error in"=w640, "fullOnly"=w637, "length"=w641, "Channel"=w642) -> ("error out"=w639:T16, "scanData"=w638:sgl[][][], "unitStrVal"=w636:string)  [unwired: 3 in, 2 out]
            }
          }
        }
        "Array" <- w612
        "ScanUnits" <- w609
        n360 = Unbundle By Name(w621) -> ("status"=w615:bool)
        n361 = local read "Stop"() -> (w614:bool)
        n362 = Compound Arithmetic op=OR(w615, w614) -> (w611:bool)
      }
      frame "promt User" {
        n363 = case shown="False" "Auto-save" {
          tunnel: [w653 Scanner_State_Machine."save" ("Enum 2")] -> w649
          frame False {
            n364 = Two Button Dialog(message="Do you want to save the measured data?", 1:"no" ("F button name (\"Cancel\")"), 2:"yes" ("T button name (\"OK\")")) -> (T button?=w655:bool)
            n365 = Select(t=Scanner_State_Machine."save" ("Enum 2"), s=w655, f=Scanner_State_Machine."wait till start" ("Enum 2")) -> (s? t:f=w653:T4)
          }
          frame True {
          }
        }
        n366 = Unbundle By Name(w643) -> ("status"=w647:bool)
        n367 = local read "Stop"() -> (w645:bool)
        n368 = Compound Arithmetic op=OR(w647, w645) -> (w644:bool)
      }
      frame "save" {
        w661 = FALSE ("Stop 2")
        n369 = local read "Corresponding channels Scan"() -> (w660:i32[])
        n370 = local read "storage paths"() -> (w659:string[])
        n371 = call "writeMultiBuffer.vi"("Corresponding channels"=w660, "storage paths"=w659, "comment"="comment", "binary"="binary", "fwd&bwd?"=TRUE, "error in"=w665) -> ("error out"=w664:T16)  [unwired: 13 in]
      }
    }
    n372 = local read "ErrorStop"() -> (w510:bool)
    n373 = case shown="True" w514 {
      tunnel: [w520 Scanner_State_Machine."wait till start" ("Enum")] -> w515
      tunnel: w516 -> [w520 _]
      frame False {
      }
      frame True {
      }
    }
    "Enum" <- w515
    n374 = Unbundle By Name(w512) -> ("status"=w517:bool)
    n375 = call "getXYPos.vi"("error in"=w512) -> ("error out"=w506:T16, "y"=→"y-position":dbl, "x"=→"x-position":dbl)  [unwired: 8 in]
    n376 = local read "Stop"() -> (w511:bool)
    n377 = Compound Arithmetic op=OR(w517, w513, w511, w510) -> (w509:bool)
    "ErrCrt_Scan" <- w509
  }
  n378 = local read "Corresponding channels"() -> (w12:i32[])
  n379 = for {
    shift-right: [w668] -> w31
    shift-left: w13 -> [w669]
    tunnel: w12 -> [w667] mode=indexing
    n380 = call "DeregDataChannel.vi"("channel"=w667, "error in"=w669) -> ("error out"=w668:T16)  [unwired: 17 in]
  }
  n381 = call "StartScan.vi"("error in"=w19, "State"=0) -> ("error out"=w18:T16)  [unwired: 9 in]
  n382 = Merge Errors(w32, w18, w31, w29) -> (w17:errorcluster)
  n383 = flat-sequence {
    tunnel: w17 -> [w671]
    tunnel: [w671] -> w16
    frame #0 {
      w670 = FALSE ("Stop")
      n384 = local write "ErrCrt_Scan"(w670) -> ()
      n385 = local write "ErrCrt_Spec"(w670) -> ()
      n386 = property on="Stop" class="Bool (strict)"("Value"=w670) -> ()  [unwired: 2 in, 2 out]
      n387 = property on="ErrCrt_Scan" class="Bool (strict)"("Value"=w670) -> ()  [unwired: 2 in, 2 out]
      n388 = local write "ErrCrt_Line"(w670) -> ()
      n389 = property on="ErrorStop" class="Bool (strict)"("Value"=w670) -> ()  [unwired: 2 in, 2 out]
    }
  }
  n390 = call "ShutdownServerCon.vi"("error in"=w16) -> ("error out"=→"error out":T16)  [unwired: 18 in]
